vi "commander10.vi"() -> ()   [LabVIEW 2015]
uses:
  <vilib>/National Instruments/NI Dynamixel API/Dynamixel Pro Driver/Controls/Write Select Pro.ctl
  <vilib>/National Instruments/NI Dynamixel API/Dynamixel Pro Driver/Controls/Baudrate Selector.ctl
  G_LCM.vi
  G_ALL.vi
  G_SEN.vi
  <vilib>/National Instruments/NI Dynamixel API/Dynamixel Pro Driver/Write/Write Dynamixel Pro.vi
  <vilib>/National Instruments/NI Dynamixel API/Dynamixel Pro Driver/Helper VIs/Torque Disable.vi
  <vilib>/National Instruments/NI Dynamixel API/Dynamixel Pro Driver/Helper VIs/Torque Enable.vi
  <vilib>/National Instruments/NI Dynamixel API/Dynamixel Pro Driver/Dynamixel Pro Driver.lvlib
panel:
  in  "map":bool
  in  "Path Num":i32 min=0 max=4 step=1
  out "CIPV_SPEED":dbl=25.0
  out "CIPV_dist":dbl=25.0
  in  "mission":i32
  out "size(s)":i32=1381
  in  "shift torque gain":i32
  out "robotis":refnum<visa-resource-name>
  in  "y 2":dbl=1.0
  in  "y":dbl=0.5 format="%#_13g"
  in  "dist_error_gain":dbl=0.5 format="%#_13g"
  in  "Global y shift":dbl min=-5.0 max=5.0 step=0.1
  in  "d":dbl=-3.5 format="%#_13g"
  in  "car detection":bool
  in  "Velodyne":T1(ring)=enum."Velodyne 64"
  in  "reset path":bool
  in  "shifthold":dbl=0.003
  out "count":i32=100
  out "signal":picture[](array[picture])=[bytes[7530], bytes[7530], bytes[7530], bytes[7530]]
  out "sign":picture[](array[picture])=[bytes[7530], bytes[7530], bytes[7530], bytes[7530]]
  out "trafic signal ref":picture[](array[picture])=[bytes[7530], bytes[7530], bytes[7530], bytes[7530], bytes[7530], bytes[7530]]
  out "sign ref":picture[](array[picture])=[bytes[7530], bytes[7530], bytes[7530], bytes[7530], bytes[7530], bytes[7530], bytes[7530], bytes[7530], bytes[7530], bytes[7530], bytes[7530], bytes[7530], bytes[7530]]
  in  "TTL":bool=TRUE
  out "obs shift":dbl format="%.2f"
  in  "lane keep":bool
  in  "replay":bool
  in  "Global x shift":dbl min=-5.0 max=5.0 step=1.0
  out "display":u32=33
  out "control":u32=10
  in  "lane update":bool
  in  "save lcm":bool
  out "LCM Recv Data":string
  out "GPS DATA 2":T2={"type"="None", "x_lcc"=0.0, "y_lcc"=0.0, "latdev"=0.0, "londev"=0.0, "sats"=0, "gps_l1_ranges"=0, "gps_l1_mask_ranges"=0, "gps_l2_mask_ranges"=0, "Heading"=0.0, "lon"=0.0, "lat"=0.0, "time"="09:00:00.0", "hgps"=0.0, "lag"=0.0, "MAP"=""} {"lag" format="%#_5g"; "hgps" format="%#_5g"; "lat" format="%#_11g"; "lon" format="%#_11g"; "Heading" format="%#_5g"; "latdev" format="%#_4g"; "londev" format="%#_4g"}
  in  "Obs":bool
  in  "Log":bool
  out "path":u32=10
  out "sensor":u32=27 format="%02.0f"
  out "Speed limit":dbl=10.0
  out "collision":bool
  in  "Load Path":bool
  in  "Max. Vel.":dbl=10.0 min=-5.0 max=120.0 step=5.0
  out "col":i16(graph)
  out "stop":bool
  in  "Reverse":bool
  in  "STOP":bool
  out "Waveform Chart 4":cluster{"auto":i16, "run":i16}(graph)={"auto"=1, "run"=0}
  out "Waveform Chart 3":cluster{"Steer_input":dbl, dbl, "handle":dbl}(graph)={"Steer_input"=0.0, -0.0, "handle"=nan}
  out "Waveform Chart 2":T3(graph)={"VS_des"=0.0, "VS_can"=0.0, "VS_des"=10.0}
  out "Heading":cluster{"Heading":dbl, "hgps":dbl}(graph)
  out "XY Graph 2":cluster{"Y":dbl[], "Y":dbl[]}[](graph)
  out "Gauge":cluster{dbl, dbl, dbl}(knob)={0.0, 0.0, 10.0} scale=-20.0..140.0
  out "Meter":cluster{dbl, dbl, dbl}(knob)={0.0, -0.0, nan} scale=-550.0..550.0
  out "XY Graph":cluster{"Y":dbl[], "Y":dbl[]}[](graph)=[{"Y"=[], "Y"=[]}, {"Y"=[-0.0, -0.0, -0.0, -0.0, -0.0, -0.0, -0.0, -0.0, -0.0, -0.0, -0.0, -0.0, -0.0, -0.0, -0.0, -0.0, -0.0, -0.0, -0.0, -0.0, -0.0, -0.0, -0.0, -0.0, -0.0, -0.0, -0.0, -0.0, -0.0, -0.0, -0.0], "Y"=[-4.0, -3.9, -3.8, -3.7, -3.6, -3.5, -3.4, -3.3, -3.2, -3.1, -3.0, -2.9, -2.8, -2.7, -2.5999999999999996, -2.5, -2.4, -2.3, -2.2, -2.0999999999999996, -2.0, -1.9, -1.7999999999999998, -1.6999999999999997, -1.5999999999999996, -1.5, -1.4, -1.2999999999999998, -1.1999999999999997, -1.0999999999999996, -1.0]}, {"Y"=[0.0], "Y"=[0.0]}, {"Y"=[], "Y"=[]}, {"Y"=[-0.925, -0.925, -0.925, -0.6775, -0.6775, -0.925, -0.925, -0.925, -0.925, -0.6775, -0.6775, -0.925, -0.925, -0.925, 0.9025, 0.9025, 0.9025, 0.6775, 0.6775, 0.9025, 0.9025, 0.9025, 0.9025, 0.6775, 0.6775, 0.9025, 0.9025, 0.9025, -0.925], "Y"=[-0.75, -0.224, 0.224, 0.224, -0.224, -0.224, 0.224, 2.415, 2.885, 2.885, 2.415, 2.415, 2.885, 3.5, 3.5, 2.885, 2.415, 2.415, 2.885, 2.885, 2.415, 0.224, -0.224, -0.224, 0.224, 0.224, -0.224, -0.75, -0.75]}, {"Y"=[-0.11693930899008871, -0.11530935243371389, -0.11366872898963808, -0.11201743865786128, -0.11035548143838347, -0.10868285733120467, -0.10699956633632488, -0.10530560845374409, -0.1036009836834623, -0.10188569202547951, -0.10015973347979573, -0.09842310804641094, -0.09667581572532517, -0.09491785651653842, -0.09314923042005063, -0.09136993743586189, -0.08957997756397212, -0.08777935080438137, -0.08596805715708963, -0.08414609662209688, -0.08231346919940313, -0.0804701748890084, -0.07861621369091265, -0.07675158560511593, -0.07487629063161819, -0.07299032877041947, -0.07109370002151975, -0.06918640438491905, -0.06726844186061733, -0.06533981244861461, -0.06340051614891093, -0.061450552961506213, -0.05948992288640052, -0.05751862592359382, -0.055536662073086135, -0.05354403133487746, -0.05154073370896778, -0.0495267691953571, -0.04750213779404542, -0.045466839505032754, -0.04342087432831909, -0.04136424226390442, -0.03929694331178877, -0.03721897747197212, -0.035130344744454464, -0.033031045129235825, -0.03092107862631617, -0.028800445235695537, -0.02666914495737389, -0.024527177791351266, -0.02237454373762765, -0.02021124279620301, -0.018037274967077403, -0.015852640250250776, -0.013657338645723171, -0.011451370153494574, -0.009234734773564957, -0.007007432505934365, -0.004769463350602757, -0.002520827307570167, -0.0002615243768365888, 0.0020084454415980058, 0.004289082147733582, 0.0065803857415701675, 0.008882356223107735, 0.011194993592346297, 0.013518297849285876, 0.01585226899392643, 0.018196907026268, 0.020552211946310545, 0.02291818375405409, 0.025294822449498655, 0.02768212803264418, 0.03008010050349072, 0.03248873986203825, 0.03490804610828678, 0.037338019242236314, 0.03977865926388684, 0.04222996617323836, 0.044691939970290875, 0.04716458065504438, 0.04964788822749888, 0.05214186268765442, 0.05464650403551091, 0.057161812271068396, 0.05968778739432688, 0.06222442940528636, 0.06477173830394688, 0.06732971409030836, 0.06989835676437083, 0.07247766632613428, 0.07506764277559874, 0.07766828611276426, 0.08027959633763071, 0.08290157345019813, 0.08553421745046658, 0.08817752833843606, 0.09083150611410651, 0.09349615077747794, 0.09617146232855037, 0.0988574407673238], "Y"=[-4.0, -3.9, -3.8, -3.7, -3.6, -3.5, -3.4, -3.3, -3.2, -3.1, -3.0, -2.9, -2.8, -2.7, -2.5999999999999996, -2.5, -2.4, -2.3, -2.2, -2.0999999999999996, -2.0, -1.9, -1.7999999999999998, -1.6999999999999997, -1.5999999999999996, -1.5, -1.4, -1.2999999999999998, -1.1999999999999997, -1.0999999999999996, -1.0, -0.8999999999999999, -0.7999999999999998, -0.6999999999999997, -0.5999999999999996, -0.5, -0.3999999999999999, -0.2999999999999998, -0.19999999999999973, -0.09999999999999964, 0.0, 0.10000000000000053, 0.20000000000000018, 0.2999999999999998, 0.40000000000000036, 0.5, 0.6000000000000005, 0.7000000000000002, 0.8000000000000007, 0.9000000000000004, 1.0, 1.1000000000000005, 1.2000000000000002, 1.3000000000000007, 1.4000000000000004, 1.5, 1.6000000000000005, 1.7000000000000002, 1.8000000000000007, 1.9000000000000004, 2.0, 2.1000000000000005, 2.2, 2.3000000000000007, 2.4000000000000004, 2.5, 2.6000000000000005, 2.7, 2.8000000000000007, 2.9000000000000004, 3.0, 3.1000000000000005, 3.2, 3.3000000000000007, 3.4000000000000004, 3.5, 3.6000000000000005, 3.7, 3.8000000000000007, 3.9000000000000004, 4.0, 4.1, 4.200000000000001, 4.300000000000001, 4.4, 4.5, 4.6, 4.700000000000001, 4.800000000000001, 4.9, 5.0, 5.1, 5.200000000000001, 5.300000000000001, 5.4, 5.5, 5.600000000000001, 5.700000000000001, 5.800000000000001, 5.9, 6.0]}, {"Y"=[0.8254985256386238, 0.8528194590155173, 0.8796538166129886, 0.9060015984310377, 0.9318628044696647, 0.9572374347288698, 0.9821254892086528, 1.0065269679090136, 1.0304418708299523, 1.0538701979714689, 1.0768119493335635, 1.099267124916236, 1.1212357247194864, 1.1427177487433147, 1.163713196987721, 1.184222069452705, 1.204244366138267, 1.2237800870444069, 1.2428292321711245, 1.2613918015184205, 1.279467795086294, 1.2970572128747455, 1.314160054883775, 1.3307763211133825, 1.3469060115635676, 1.3625491262343308, 1.3777056651256718, 1.392375628237591, 1.4065590155700878, 1.4202558271231627, 1.4334660628968152, 1.4461897228910459, 1.4584268071058544, 1.4701773155412408, 1.4814412481972052, 1.4922186050737474, 1.5025093861708676, 1.5123135914885657, 1.5216312210268417, 1.5304622747856955, 1.5388067527651272, 1.546664654965137, 1.5540359813857245, 1.56092073202689, 1.5673189068886335, 1.5732305059709548, 1.578655529273854, 1.583593976797331, 1.5880458485413862, 1.592011144506019, 1.5954898646912299, 1.5984820090970187, 1.6009875777233853, 1.60300657057033, 1.6045389876378524, 1.605584828925953, 1.606144094434631, 1.6062167841638872, 1.6058028981137213, 1.6049024362841335, 1.6035153986751234, 1.601641785286691, 1.599281596118837, 1.5964348311715606, 1.5931014904448622, 1.5892815739387416, 1.584975081653199, 1.5801820135882343, 1.5749023697438473, 1.5691361501200385, 1.5628833547168075, 1.5561439835341544, 1.5489180365720792, 1.541205513830582, 1.5330064153096625, 1.5243207410093211, 1.5151484909295576, 1.505489665070372, 1.4953442634317642, 1.4847122860137343, 1.4735937328162825, 1.4619886038394085, 1.4498968990831123, 1.437318618547394, 1.4242537622322538, 1.4107023301376915, 1.396664322263707, 1.3821397386103003, 1.3671285791774717, 1.351630843965221, 1.335646532973548, 1.3191756462024533, 1.302218183651936, 1.284774145321997, 1.2668435312126356, 1.2484263413238526, 1.229522575655647, 1.2101322342080194, 1.19025531698097, 1.1698918239744982, 1.1490417551886045], "Y"=[-4.0, -3.9, -3.8, -3.7, -3.6, -3.5, -3.4, -3.3, -3.2, -3.1, -3.0, -2.9, -2.8, -2.7, -2.5999999999999996, -2.5, -2.4, -2.3, -2.2, -2.0999999999999996, -2.0, -1.9, -1.7999999999999998, -1.6999999999999997, -1.5999999999999996, -1.5, -1.4, -1.2999999999999998, -1.1999999999999997, -1.0999999999999996, -1.0, -0.8999999999999999, -0.7999999999999998, -0.6999999999999997, -0.5999999999999996, -0.5, -0.3999999999999999, -0.2999999999999998, -0.19999999999999973, -0.09999999999999964, 0.0, 0.10000000000000053, 0.20000000000000018, 0.2999999999999998, 0.40000000000000036, 0.5, 0.6000000000000005, 0.7000000000000002, 0.8000000000000007, 0.9000000000000004, 1.0, 1.1000000000000005, 1.2000000000000002, 1.3000000000000007, 1.4000000000000004, 1.5, 1.6000000000000005, 1.7000000000000002, 1.8000000000000007, 1.9000000000000004, 2.0, 2.1000000000000005, 2.2, 2.3000000000000007, 2.4000000000000004, 2.5, 2.6000000000000005, 2.7, 2.8000000000000007, 2.9000000000000004, 3.0, 3.1000000000000005, 3.2, 3.3000000000000007, 3.4000000000000004, 3.5, 3.6000000000000005, 3.7, 3.8000000000000007, 3.9000000000000004, 4.0, 4.1, 4.200000000000001, 4.300000000000001, 4.4, 4.5, 4.6, 4.700000000000001, 4.800000000000001, 4.9, 5.0, 5.1, 5.200000000000001, 5.300000000000001, 5.4, 5.5, 5.600000000000001, 5.700000000000001, 5.800000000000001, 5.9, 6.0]}, {"Y"=[-1.0593771436188013, -1.0834381638829451, -1.1069912745922648, -1.1300364757467602, -1.1525737673464316, -1.1746031493912792, -1.1961246218813026, -1.2171381848165017, -1.2376438381968768, -1.257641582022428, -1.277131416293155, -1.296113341009058, -1.314587356170137, -1.3325534617763914, -1.3500116578278223, -1.3669619443244287, -1.3834043212662113, -1.3993387886531696, -1.4147653464853038, -1.4296839947626143, -1.4440947334851004, -1.4579975626527624, -1.4713924822656004, -1.4842794923236142, -1.4966585928268041, -1.5085297837751699, -1.5198930651687115, -1.530748437007429, -1.5410958992913224, -1.5509354520203917, -1.5602670951946371, -1.5690908288140584, -1.5774066528786554, -1.5852145673884286, -1.5925145723433776, -1.5993066677435024, -1.605590853588803, -1.6113671298792798, -1.6166354966149326, -1.621395953795761, -1.6256485014217654, -1.6293931394929457, -1.632629868009302, -1.6353586869708343, -1.6375795963775424, -1.6392925962294265, -1.6404976865264864, -1.6411948672687222, -1.6413841384561338, -1.6410655000887215, -1.6402389521664853, -1.6389044946894247, -1.6370621276575401, -1.6347118510708316, -1.6318536649292987, -1.628487569232942, -1.624613563981761, -1.620231649175756, -1.615341824814927, -1.6099440908992737, -1.6040384474287965, -1.5976248944034952, -1.5907034318233697, -1.5832740596884203, -1.5753367779986467, -1.566891586754049, -1.5579384859546273, -1.5484774756003814, -1.5385085556913114, -1.5280317262274175, -1.5170469872086993, -1.505554338635157, -1.4935537805067909, -1.4810453128236005, -1.4680289355855862, -1.4545046487927475, -1.440472452445085, -1.4259323465425984, -1.4108843310852874, -1.3953284060731526, -1.3792645715061937, -1.3626928273844108, -1.3456131737078034, -1.3280256104763721, -1.309930137690117, -1.2913267553490377, -1.2722154634531344, -1.2525962620024065, -1.232469150996855, -1.2118341304364795, -1.1906912003212795, -1.1690403606512558, -1.1468816114264073, -1.1242149526467355, -1.1010403843122396, -1.077357906422919, -1.0531675189787748, -1.0284692219798064, -1.0032630154260138, -0.9775488993173974, -0.9513268736539569], "Y"=[-4.0, -3.9, -3.8, -3.7, -3.6, -3.5, -3.4, -3.3, -3.2, -3.1, -3.0, -2.9, -2.8, -2.7, -2.5999999999999996, -2.5, -2.4, -2.3, -2.2, -2.0999999999999996, -2.0, -1.9, -1.7999999999999998, -1.6999999999999997, -1.5999999999999996, -1.5, -1.4, -1.2999999999999998, -1.1999999999999997, -1.0999999999999996, -1.0, -0.8999999999999999, -0.7999999999999998, -0.6999999999999997, -0.5999999999999996, -0.5, -0.3999999999999999, -0.2999999999999998, -0.19999999999999973, -0.09999999999999964, 0.0, 0.10000000000000053, 0.20000000000000018, 0.2999999999999998, 0.40000000000000036, 0.5, 0.6000000000000005, 0.7000000000000002, 0.8000000000000007, 0.9000000000000004, 1.0, 1.1000000000000005, 1.2000000000000002, 1.3000000000000007, 1.4000000000000004, 1.5, 1.6000000000000005, 1.7000000000000002, 1.8000000000000007, 1.9000000000000004, 2.0, 2.1000000000000005, 2.2, 2.3000000000000007, 2.4000000000000004, 2.5, 2.6000000000000005, 2.7, 2.8000000000000007, 2.9000000000000004, 3.0, 3.1000000000000005, 3.2, 3.3000000000000007, 3.4000000000000004, 3.5, 3.6000000000000005, 3.7, 3.8000000000000007, 3.9000000000000004, 4.0, 4.1, 4.200000000000001, 4.300000000000001, 4.4, 4.5, 4.6, 4.700000000000001, 4.800000000000001, 4.9, 5.0, 5.1, 5.200000000000001, 5.300000000000001, 5.4, 5.5, 5.600000000000001, 5.700000000000001, 5.800000000000001, 5.9, 6.0]}, {"Y"=[], "Y"=[]}, {"Y"=[0.0], "Y"=[0.0]}, {"Y"=[], "Y"=[]}, {"Y"=[], "Y"=[]}, {"Y"=[0.0], "Y"=[0.0]}, {"Y"=[-2.34, -2.34, -2.34, -2.34, -2.2800000000000002, -2.2800000000000002, -2.2800000000000002, -2.2800000000000002, -2.22, -2.22, -2.22, -2.16, -2.16, -2.16, -2.1, -2.1, -2.1, -2.04, -2.04, -2.04, -2.04, -1.98, -1.98, -1.98, -1.98, -1.68, -1.68, -1.68, -1.68, -1.68, -1.68, -1.68, -1.68, -1.68, -1.68, -1.68, -1.68, -1.68, -1.68, -1.68, -1.68, -1.68, -1.68, -1.68, -1.68, -1.68, -1.68, -1.68, -1.68, -1.68, -1.68, -1.68, -1.68, -1.68, -1.68, -1.68, -1.68, -1.68, -1.68, -1.68, -1.68, -1.68, -1.68, -1.68, -1.68, -1.68, -1.68, -1.62, -1.62, -1.62, -1.62, -1.62, -1.62, -1.62, -1.62, -1.62, -1.62, -1.62, -1.62, -1.62, -1.62, -1.62, -1.62, -1.62, -1.62, -1.62, -1.62, -1.62, -1.62, -1.62, -1.62, -1.62, -1.62, -1.62, -1.62, -1.62, -1.62, -1.62, -1.62, -1.62, -1.62, -1.62, -1.62, -1.62, -1.62, -1.62, -1.62, -1.62, -1.62, -1.62, -1.62, -1.62, -1.62, -1.62, -1.62, -1.62, -1.62, -1.62, -1.62, -1.62, -1.62, -1.62, -1.62, -1.62, -1.62, -1.62, -1.62, -1.62, -1.62, -1.62, -1.62, -1.62, -1.62, -1.62, -1.62, -1.62, -1.62, -1.62, -1.62, -1.62, -1.62, -1.62, -1.62, -1.62, -1.62, -1.62, -1.62, -1.56, -1.56, -1.56, -1.56, -1.56, -1.56, -1.56, -1.56, -1.56, -1.56, -1.56, -1.56, -1.56, -1.56, -1.56, -1.56, -1.56, -1.56, -1.56, -1.56, -1.56, -1.56, -1.56, -1.56, -1.56, -1.56, -1.56, -1.56, -1.56, -1.56, -1.56, -1.56, -1.56, -1.56, -1.56, -1.56, -1.56, -1.56, -1.56, -1.56, -1.56, -1.56, -1.56, -1.56, -1.56, -1.56, -1.56, -1.56, -1.56, -1.56, -1.56, -1.56, -1.56, -1.56, -1.56, -1.56, -1.56, -1.56, -1.56, -1.56, -1.56, -1.56, -1.56, -1.56, -1.56, -1.56, -1.56, -1.56, -1.56, -1.56, -1.56, -1.56, -1.56, -1.56, -1.56, -1.56, -1.56, -1.56, -1.56, -1.56, -1.56, -1.56, -1.56, -1.56, -1.56, -1.56, -1.56, -1.56, -1.56, -1.56, -1.56, -1.56, -1.56, -1.56, -1.5, -1.5, -1.5, -1.5, -1.5, -1.5, -1.5, -1.5, -1.5, -1.5, -1.5, -1.5, -1.5, -1.5, -1.5, -1.5, -1.5, -1.5, -1.5, -1.5, -1.5, -1.5, -1.5, -1.5, -1.5, -1.5, -1.5, -1.5, -1.5, -1.5, -1.5, -1.5, -1.5, -1.5, -1.5, -1.5, -1.5, -1.5, -1.5, -1.5, -1.5, -1.5, -1.5, -1.5, -1.5, -1.5, -1.5, -1.5, -1.5, -1.5, -1.44, -1.44, -1.44, -1.44, -1.44, -1.44, -1.44, -1.44, -1.44, -1.44, -1.44, -1.44, -1.44, -1.44, -1.44, -1.44, -1.44, -1.44, -1.44, -1.44, -1.44, -1.44, -1.44, -1.44, -1.44, -1.44, -1.44, -1.44, -1.44, -1.44, -1.44, -1.44, -1.44, -1.44, -1.3800000000000001, -1.3800000000000001, -1.3800000000000001, -1.3800000000000001, -1.3800000000000001, -1.3800000000000001, -1.3800000000000001, -1.3800000000000001, -1.3800000000000001, -1.3800000000000001, -1.3800000000000001, -1.3800000000000001, -1.3800000000000001, -1.3800000000000001, -1.3800000000000001, -1.3800000000000001, -1.3800000000000001, -1.3800000000000001, -1.3800000000000001, -1.3800000000000001, -1.3800000000000001, -1.32, -1.32, -1.32, -1.32, -1.32, -1.32, -1.32, -1.32, -1.32, -1.32, -1.32, -1.32, -1.32, -1.32, -1.32, -1.32, -1.32, -1.32, -1.32, -1.32, -1.32, -1.26, -1.26, -1.26, -1.26, -1.26, -1.26, -1.26, -1.26, -1.26, -1.26, -1.26, -1.26, -1.26, -1.26, -1.26, -1.26, -1.26, -1.26, -1.26, -1.26, -1.26, -1.26, -1.26, -1.26, -1.26, -1.26, -1.26, -1.26, -1.2, -1.2, -1.2, -1.2, -1.2, -1.2, -1.2, -1.2, -1.2, -1.2, -1.2, -1.2, -1.2, -1.2, -1.2, -1.2, -1.2, -1.2, -1.2, -1.2, -1.2, -1.2, -1.2, -1.2, -1.2, -1.2, -1.2, -1.2, -1.2, -1.1400000000000001, -1.1400000000000001, -1.1400000000000001, -1.1400000000000001, -1.1400000000000001, -1.1400000000000001, -1.1400000000000001, -1.1400000000000001, -1.1400000000000001, -1.1400000000000001, -1.1400000000000001, -1.1400000000000001, -1.1400000000000001, -1.1400000000000001, -1.1400000000000001, -1.1400000000000001, -1.1400000000000001, -1.1400000000000001, -1.1400000000000001, -1.1400000000000001, -1.1400000000000001, -1.1400000000000001, -1.1400000000000001, -1.1400000000000001, -1.1400000000000001, -1.1400000000000001, -1.1400000000000001, -1.08, -1.08, -1.08, -1.08, -1.08, -1.08, -1.08, -1.08, -1.08, -1.08, -1.08, -1.08, -1.08, -1.08, -1.08, -1.08, -1.08, -1.08, -1.08, -1.08, -1.08, -1.02, -1.02, -1.02, -1.02, -1.02, -1.02, -1.02, -1.02, -1.02, -1.02, -1.02, -1.02, -1.02, -1.02, -1.02, -1.02, -1.02, -1.02, -1.02, -1.02, -0.96, -0.96, -0.96, -0.96, -0.96, -0.96, -0.96, -0.96, -0.96, -0.96, -0.96, -0.96, -0.96, -0.96, -0.96, -0.96, -0.96, -0.96, -0.96, -0.96, -0.96, -0.96, -0.96, -0.96, -0.96, -0.96, -0.9, -0.9, -0.9, -0.9, -0.9, -0.9, -0.9, -0.9, -0.9, -0.9, -0.9, -0.9, -0.9, -0.9, -0.9, -0.9, -0.9, -0.9, -0.9, -0.9, -0.9, -0.9, -0.9, -0.9, -0.9, -0.9, -0.9, -0.84, -0.84, -0.84, -0.84, -0.84, -0.84, -0.84, -0.84, -0.84, -0.84, -0.84, -0.84, -0.84, -0.84, -0.84, -0.84, -0.84, -0.84, -0.84, -0.84, -0.84, -0.84, -0.84, -0.84, -0.84, -0.84, -0.84, -0.78, -0.78, -0.78, -0.78, -0.78, -0.78, -0.78, -0.78, -0.78, -0.78, -0.78, -0.78, -0.78, -0.78, -0.78, -0.78, -0.78, -0.78, -0.78, -0.78, -0.78, -0.78, -0.78, -0.78, -0.72, -0.72, -0.72, -0.72, -0.72, -0.72, -0.72, -0.72, -0.72, -0.72, -0.72, -0.72, -0.72, -0.72, -0.72, -0.72, -0.72, -0.72, -0.72, -0.72, -0.72, -0.72, -0.66, -0.66, -0.66, -0.66, -0.66, -0.66, -0.66, -0.66, -0.66, -0.66, -0.66, -0.66, -0.66, -0.66, -0.66, -0.66, -0.66, -0.66, -0.66, -0.66, -0.66, -0.66, -0.66, -0.66, -0.66, -0.66, -0.66, -0.66, -0.66, -0.66, -0.66, -0.66, -0.66, -0.66, -0.6, -0.6, -0.6, -0.6, -0.6, -0.6, -0.6, -0.6, -0.6, -0.6, -0.6, -0.6, -0.6, -0.6, -0.6, -0.6, -0.6, -0.6, -0.6, -0.6, -0.6, -0.6, -0.6, -0.6, -0.6, -0.6, -0.6, -0.54, -0.54, -0.54, -0.54, -0.54, -0.54, -0.54, -0.54, -0.54, -0.54, -0.54, -0.54, 0.54, 0.54, 0.54, 0.54, 0.54, 0.54, 0.54, 0.54, 0.54, 0.6, 0.6, 0.6, 0.6, 0.6, 0.6, 0.6, 0.6, 0.6, 0.6, 0.6, 0.6, 0.6, 0.66, 0.66, 0.66, 0.66, 0.66, 0.66, 0.66, 0.66, 0.66, 0.66, 0.66, 0.66, 0.66, 0.66, 0.72, 0.72, 0.72, 0.72, 0.72, 0.72, 0.72, 0.72, 0.72, 0.78, 0.78, 0.78, 0.78, 0.78, 0.78, 0.78, 0.78, 0.78, 0.78, 0.78, 0.78, 0.84, 0.84, 0.84, 0.84, 0.84, 0.84, 0.84, 0.84, 0.84, 0.84, 0.84, 0.84, 0.9, 0.9, 0.9, 0.9, 0.9, 0.9, 0.9, 0.9, 0.9, 0.9, 0.9, 0.9, 0.9, 0.9, 0.9, 0.9, 0.9, 0.9, 0.9, 0.9, 0.96, 0.96, 0.96, 0.96, 0.96, 0.96, 0.96, 0.96, 0.96, 0.96, 0.96, 0.96, 0.96, 0.96, 0.96, 0.96, 0.96, 0.96, 0.96, 0.96, 0.96, 0.96, 0.96, 0.96, 0.96, 0.96, 0.96, 0.96, 1.02, 1.02, 1.02, 1.02, 1.02, 1.02, 1.02, 1.02, 1.02, 1.02, 1.02, 1.02, 1.02, 1.02, 1.02, 1.02, 1.02, 1.02, 1.02, 1.02, 1.02, 1.02, 1.02, 1.02, 1.02, 1.02, 1.02, 1.02, 1.02, 1.02, 1.02, 1.02, 1.08, 1.08, 1.08, 1.08, 1.08, 1.08, 1.08, 1.08, 1.08, 1.08, 1.08, 1.08, 1.08, 1.08, 1.08, 1.08, 1.08, 1.08, 1.08, 1.08, 1.08, 1.08, 1.08, 1.08, 1.08, 1.08, 1.08, 1.08, 1.08, 1.08, 1.08, 1.08, 1.08, 1.08, 1.08, 1.08, 1.1400000000000001, 1.1400000000000001, 1.1400000000000001, 1.1400000000000001, 1.1400000000000001, 1.1400000000000001, 1.1400000000000001, 1.1400000000000001, 1.1400000000000001, 1.1400000000000001, 1.1400000000000001, 1.1400000000000001, 1.1400000000000001, 1.1400000000000001, 1.1400000000000001, 1.1400000000000001, 1.1400000000000001, 1.1400000000000001, 1.1400000000000001, 1.1400000000000001, 1.1400000000000001, 1.1400000000000001, 1.1400000000000001, 1.1400000000000001, 1.1400000000000001, 1.1400000000000001, 1.1400000000000001, 1.1400000000000001, 1.1400000000000001, 1.1400000000000001, 1.1400000000000001, 1.1400000000000001, 1.1400000000000001, 1.1400000000000001, 1.1400000000000001, 1.1400000000000001, 1.1400000000000001, 1.2, 1.2, 1.2, 1.2, 1.2, 1.2, 1.2, 1.2, 1.2, 1.2, 1.2, 1.2, 1.2, 1.2, 1.2, 1.2, 1.2, 1.2, 1.2, 1.2, 1.2, 1.2, 1.2, 1.2, 1.2, 1.2, 1.2, 1.2, 1.2, 1.26, 1.26, 1.26, 1.26, 1.26, 1.26, 1.26, 1.26, 1.26, 1.26, 1.26, 1.26, 1.26, 1.26, 1.26, 1.26, 1.26, 1.26, 1.26, 1.26, 1.26, 1.26, 1.26, 1.26, 1.26, 1.26, 1.26, 1.26, 1.26, 1.26, 1.26, 1.26, 1.26, 1.26, 1.32, 1.32, 1.32, 1.32, 1.32, 1.32, 1.32, 1.32, 1.32, 1.32, 1.32, 1.32, 1.32, 1.32, 1.32, 1.32, 1.32, 1.32, 1.32, 1.32, 1.32, 1.32, 1.32, 1.32, 1.32, 1.32, 1.32, 1.32, 1.32, 1.32, 1.32, 1.32, 1.32, 1.32, 1.32, 1.3800000000000001, 1.3800000000000001, 1.3800000000000001, 1.3800000000000001, 1.3800000000000001, 1.3800000000000001, 1.3800000000000001, 1.3800000000000001, 1.3800000000000001, 1.3800000000000001, 1.3800000000000001, 1.3800000000000001, 1.3800000000000001, 1.3800000000000001, 1.3800000000000001, 1.3800000000000001, 1.3800000000000001, 1.3800000000000001, 1.3800000000000001, 1.3800000000000001, 1.3800000000000001, 1.3800000000000001, 1.3800000000000001, 1.3800000000000001, 1.3800000000000001, 1.3800000000000001, 1.3800000000000001, 1.3800000000000001, 1.3800000000000001, 1.3800000000000001, 1.3800000000000001, 1.3800000000000001, 1.3800000000000001, 1.3800000000000001, 1.3800000000000001, 1.44, 1.44, 1.44, 1.44, 1.44, 1.44, 1.44, 1.44, 1.44, 1.44, 1.44, 1.44, 1.44, 1.44, 1.44, 1.44, 1.44, 1.44, 1.44, 1.44, 1.44, 1.44, 1.44, 1.44, 1.44, 1.44, 1.44, 1.44, 1.44, 1.44, 1.44, 1.44, 1.44, 1.44, 1.44, 1.44, 1.44, 1.44, 1.44, 1.44, 1.5, 1.5, 1.5, 1.5, 1.5, 1.5, 1.5, 1.5, 1.5, 1.5, 1.5, 1.5, 1.5, 1.5, 1.5, 1.5, 1.5, 1.5, 1.5, 1.5, 1.5, 1.5, 1.5, 1.5, 1.5, 1.5, 1.5, 1.5, 1.5, 1.5, 1.5, 1.5, 1.5, 1.5, 1.5, 1.5, 1.5, 1.5, 1.5, 1.5, 1.5, 1.5, 1.5, 1.5, 1.5, 1.5, 1.5, 1.5, 1.5, 1.5, 1.5, 1.5, 1.5, 1.5, 1.5, 1.5, 1.5, 1.5, 1.5, 1.5, 1.5, 1.5, 1.5, 1.56, 1.56, 1.56, 1.56, 1.56, 1.56, 1.56, 1.56, 1.56, 1.56, 1.56, 1.56, 1.56, 1.56, 1.56, 1.56, 1.56, 1.56, 1.56, 1.56, 1.56, 1.56, 1.56, 1.56, 1.56, 1.56, 1.56, 1.56, 1.56, 1.56, 1.56, 1.56, 1.56, 1.56, 1.56, 1.56, 1.56, 1.56, 1.56, 1.56, 1.56, 1.56, 1.56, 1.56, 1.56, 1.56, 1.56, 1.56, 1.56, 1.56, 1.56, 1.56, 1.56, 1.56, 1.56, 1.56, 1.56, 1.56, 1.56, 1.56, 1.56, 1.56, 1.56, 1.56, 1.56, 1.56, 1.56, 1.56, 1.56, 1.56, 1.56, 1.56, 1.56, 1.56, 1.56, 1.56, 1.56, 1.56, 1.56, 1.56, 1.56, 1.56, 1.56, 1.56, 1.56, 1.62, 1.62, 1.62, 1.62, 1.62, 1.62, 1.62, 1.62, 1.62, 1.62, 1.62, 1.62, 1.62, 1.62, 1.62, 1.62, 1.62, 1.62, 1.62, 1.62, 1.62, 1.62, 1.62, 1.62, 1.62, 1.62, 1.62, 1.62, 1.62, 1.62, 1.62, 1.62, 1.62, 1.62, 1.62, 1.62, 1.62, 1.62, 1.62, 1.62, 1.62, 1.62, 1.62, 1.62, 1.62, 1.62, 1.62, 1.62, 1.62, 1.62, 1.62, 1.62, 1.62, 1.62, 1.62, 1.62, 1.62, 1.62, 1.62, 1.62, 1.62, 1.62, 1.62, 1.62, 1.62, 1.62, 1.62, 1.62, 1.62, 1.62, 1.62, 1.62, 1.68, 1.68, 1.68, 1.68, 1.68, 1.68, 1.68, 1.68, 1.68, 1.68, 1.68, 1.68, 1.68, 1.68, 1.74, 1.74, 1.74, 1.74, 1.74, 1.8, 1.8, 1.8, 1.8, 1.8, 1.8, 1.86, 1.86, 1.86, 1.86, 1.92, 1.92, 1.92, 1.92, 1.92, 1.98, 1.98, 1.98, 1.98, 1.98, 1.98, 2.04, 2.04, 2.04, 2.04, 2.04, 2.1, 2.1, 2.1, 2.1, 2.1, 2.16, 2.16, 2.16, 2.16, 2.22, 2.22, 2.22, 2.22, 2.2800000000000002, 2.2800000000000002, 2.2800000000000002, 2.2800000000000002, 2.2800000000000002, 2.2800000000000002, 2.2800000000000002, 2.34, 2.34, 2.34, 2.34, 2.34, 2.34, 2.34, 2.34, 2.34, 2.34], "Y"=[-5.88, -5.94, -6.0, -6.0600000000000005, -5.88, -5.94, -6.0, -6.0600000000000005, -5.88, -5.94, -6.0, -6.3, -6.36, -6.42, -6.3, -6.36, -6.42, -6.24, -6.3, -6.36, -6.42, -6.24, -6.3, -6.36, -6.42, 2.04, 1.98, 1.92, 1.86, 1.8, 1.74, 1.68, 1.62, 1.56, 1.5, 1.3800000000000001, 1.32, 1.26, 1.2, 1.1400000000000001, 1.08, 1.02, 0.96, 0.9, 0.84, 0.78, 0.72, 0.66, 0.6, 0.54, 0.48, 0.42, 0.36, 0.3, 0.24, 0.18, 0.12, 0.06, -0.0, -0.06, -0.12, -0.18, -0.24, -0.3, -0.36, -0.42, -0.48, 3.24, 3.18, 3.12, 3.06, 3.0, 2.94, 2.88, 2.82, 2.7600000000000002, 2.7, 2.64, 2.58, 2.52, 2.46, 2.4, 2.34, 2.2800000000000002, 2.22, 2.16, 2.1, 2.04, 1.98, 1.92, 1.86, 1.8, 1.74, 1.68, 1.62, 1.56, 1.5, 1.44, 1.3800000000000001, 1.32, 1.26, 1.2, 1.1400000000000001, 1.08, 1.02, 0.96, 0.9, 0.84, 0.78, 0.72, 0.66, 0.6, 0.54, 0.48, 0.42, 0.36, 0.3, 0.24, 0.18, 0.12, 0.06, -0.0, -0.06, -0.12, -0.18, -0.24, -0.3, -0.36, -0.42, -0.48, -0.54, -0.6, -0.66, -0.72, -0.78, -0.84, -0.9, -0.96, -1.02, -1.08, -1.1400000000000001, -1.2, -1.26, -1.32, -1.3800000000000001, -1.44, -1.5, 3.72, 3.66, 3.6, 3.54, 3.48, 3.42, 3.36, 3.3000000000000003, 3.24, 3.18, 3.12, 3.06, 3.0, 2.94, 2.88, 2.82, 2.7600000000000002, 2.7, 2.64, 2.58, 2.52, 2.46, 2.4, 2.34, 2.2800000000000002, 2.22, 2.16, 2.1, 2.04, 1.98, 1.92, 1.86, 1.8, 1.74, 1.68, 1.62, 1.56, 1.5, 1.44, 1.3800000000000001, 1.32, 1.26, 1.2, 1.1400000000000001, 1.08, 1.02, 0.96, 0.9, 0.84, 0.78, 0.72, 0.66, 0.6, 0.54, 0.48, 0.42, 0.36, 0.3, 0.24, 0.18, 0.12, 0.06, -0.0, -0.06, -0.12, -0.18, -0.24, -0.3, -0.36, -0.42, -0.48, -0.54, -0.6, -0.66, -0.72, -0.78, -0.84, -0.9, -0.96, -1.02, -1.08, -1.1400000000000001, -1.2, -1.26, -1.32, -1.3800000000000001, -1.44, -1.5, -1.56, -1.62, -1.68, -1.74, -1.8, -1.86, 3.72, 3.66, 3.6, 3.54, 3.48, 3.42, 3.36, 3.3000000000000003, 3.24, 3.18, 3.12, 3.06, 3.0, 2.94, 2.88, 2.82, 2.7600000000000002, 2.7, 2.64, 2.58, 2.52, 2.46, 2.4, 2.34, -0.54, -0.6, -0.66, -0.84, -0.9, -0.96, -1.02, -1.08, -1.1400000000000001, -1.2, -1.26, -1.32, -1.3800000000000001, -1.44, -1.5, -1.56, -1.62, -1.68, -1.74, -1.8, -1.86, -1.92, -1.98, -2.04, -2.1, -2.16, 3.96, 3.9, 3.84, 3.7800000000000002, 3.72, 3.66, 3.6, 3.54, 3.48, 3.42, 3.36, 3.3000000000000003, 3.24, 3.18, 3.12, -1.44, -1.5, -1.56, -1.62, -1.68, -1.74, -1.8, -1.86, -1.92, -1.98, -2.04, -2.1, -2.16, -2.22, -2.2800000000000002, -2.34, -2.4, -2.46, -2.52, 4.2, 4.14, 4.08, 4.0200000000000005, 3.96, 3.9, 3.84, 3.7800000000000002, 3.72, 3.66, -1.98, -2.04, -2.1, -2.16, -2.22, -2.2800000000000002, -2.34, -2.4, -2.46, -2.52, -2.58, 4.5600000000000005, 4.5, 4.44, 4.38, 4.32, 4.26, 4.2, 4.14, 4.08, 4.0200000000000005, 3.96, -2.34, -2.4, -2.46, -2.52, -2.58, -2.64, -2.7, -2.7600000000000002, -2.82, -2.88, 4.92, 4.86, 4.8, 4.74, 4.68, 4.62, 4.5600000000000005, 4.5, 4.44, 4.38, 4.32, 4.26, 4.2, -2.52, -2.58, -2.64, -2.7, -2.7600000000000002, -2.82, -2.88, -2.94, -3.0, -3.06, -3.12, -3.18, -3.24, -3.3000000000000003, -3.36, 5.16, 5.1000000000000005, 5.04, 4.98, 4.92, 4.86, 4.8, 4.74, 4.68, 4.62, 4.5600000000000005, 4.5, 4.44, 4.38, -2.94, -3.0, -3.06, -3.12, -3.18, -3.24, -3.3000000000000003, -3.36, -3.42, -3.48, -3.54, -3.6, -3.66, -3.72, -3.7800000000000002, 5.64, 5.58, 5.5200000000000005, 5.46, 5.4, 5.34, 5.28, 5.22, 5.16, 5.1000000000000005, 5.04, 4.98, 4.92, 4.86, 4.8, -3.36, -3.42, -3.48, -3.54, -3.6, -3.66, -3.72, -3.7800000000000002, -3.84, -3.9, -3.96, -4.0200000000000005, 6.0, 5.94, 5.88, 5.82, 5.76, 5.7, 5.64, 5.58, 5.5200000000000005, 5.46, 5.4, 5.34, 5.28, 5.22, -3.84, -3.9, -3.96, -4.0200000000000005, -4.08, -4.14, -4.2, 6.24, 6.18, 6.12, 6.0600000000000005, 6.0, 5.94, 5.88, 5.82, 5.76, 5.7, 5.64, 5.58, 5.5200000000000005, -4.14, -4.2, -4.26, -4.32, -4.38, -4.44, -4.5, 6.72, 6.66, 6.6000000000000005, 6.54, 6.48, 6.42, 6.36, 6.3, 6.24, 6.18, 6.12, 6.0600000000000005, 6.0, 5.94, -4.2, -4.26, -4.32, -4.38, -4.44, -4.5, -4.5600000000000005, -4.62, -4.68, -4.74, -4.8, -4.86, 7.2, 7.140000000000001, 7.08, 7.0200000000000005, 6.96, 6.9, 6.84, 6.78, 6.72, 6.66, 6.6000000000000005, 6.54, 6.48, 6.42, 6.36, 6.3, -4.44, -4.5, -4.5600000000000005, -4.62, -4.68, -4.74, -4.8, -4.86, -4.92, -4.98, -5.04, 7.5600000000000005, 7.5, 7.44, 7.38, 7.32, 7.26, 7.2, 7.140000000000001, 7.08, 7.0200000000000005, 6.96, 6.9, 6.84, 6.78, 6.72, 6.66, 6.6000000000000005, -4.74, -4.8, -4.86, -4.92, -4.98, -5.04, -5.1000000000000005, -5.16, -5.22, -5.28, 7.86, 7.8, 7.74, 7.68, 7.62, 7.5600000000000005, 7.5, 7.44, 7.38, 7.32, 7.26, 7.2, 7.140000000000001, 7.08, 7.0200000000000005, -4.98, -5.04, -5.1000000000000005, -5.16, -5.22, -5.28, -5.34, -5.4, -5.46, 7.98, 7.92, 7.86, 7.8, 7.74, 7.68, 7.62, 7.5600000000000005, 7.5, -5.04, -5.1000000000000005, -5.16, -5.22, -5.28, -5.34, -5.4, -5.46, -5.5200000000000005, -5.58, -5.64, -5.7, -5.76, 8.46, 8.4, 8.34, 8.28, 8.22, 8.16, 8.1, 8.040000000000001, 7.98, 7.92, 7.86, 7.8, 7.74, 7.68, 7.62, -5.22, -5.28, -5.34, -5.4, -5.46, -5.5200000000000005, -5.58, -5.64, -5.7, -5.76, -5.82, -5.88, -5.94, -6.0, -6.0600000000000005, -6.12, -6.18, -6.24, -6.3, 8.88, 8.82, 8.76, 8.700000000000001, 8.64, 8.58, 8.52, 8.46, 8.4, 8.34, 8.28, 8.22, 8.16, -5.64, -5.7, -5.76, -5.82, -5.88, -5.94, -6.0, -6.0600000000000005, -6.12, -6.18, -6.24, -6.3, -6.36, -6.42, 8.88, 8.82, 8.76, 8.52, 8.46, -6.0600000000000005, -6.12, -6.18, -6.24, -6.3, -6.36, -6.42, -5.16, -5.22, -5.28, -5.34, -5.4, -5.46, -5.5200000000000005, -5.58, -5.64, -4.92, -4.98, -5.04, -5.1000000000000005, -5.16, -5.22, -5.28, -5.34, -5.4, -5.46, -5.5200000000000005, -5.58, -5.64, -4.68, -4.74, -4.8, -4.86, -4.92, -4.98, -5.04, -5.1000000000000005, -5.16, -5.22, -5.28, -5.34, -5.4, -5.46, -4.32, -4.38, -4.44, -4.5, -4.5600000000000005, -4.62, -4.68, -4.74, -4.8, -4.0200000000000005, -4.08, -4.14, -4.2, -4.26, -4.32, -4.38, -4.44, -4.5, -4.5600000000000005, -4.62, -4.68, -3.84, -3.9, -3.96, -4.0200000000000005, -4.08, -4.14, -4.2, -4.26, -4.32, -4.38, -4.44, -4.5, 9.0, 8.94, 8.88, 8.82, 8.76, 8.700000000000001, 8.64, 8.58, 8.52, 8.46, -3.54, -3.6, -3.66, -3.72, -3.7800000000000002, -3.84, -3.9, -3.96, -4.0200000000000005, -4.08, 9.0, 8.94, 8.88, 8.82, 8.76, 8.700000000000001, 8.64, 8.58, 8.52, 8.46, 7.92, 7.86, 7.8, 7.74, 7.68, 7.62, 7.5600000000000005, 7.5, -3.3000000000000003, -3.36, -3.42, -3.48, -3.54, -3.6, -3.66, -3.72, -3.7800000000000002, -3.84, 7.92, 7.86, 7.8, 7.74, 7.68, 7.62, 7.5600000000000005, 7.5, 7.44, 7.38, 7.32, 7.26, 7.2, 7.140000000000001, 7.08, 7.0200000000000005, 6.96, 6.9, 6.84, 6.78, -2.94, -3.0, -3.06, -3.12, -3.18, -3.24, -3.3000000000000003, -3.36, -3.42, -3.48, -3.54, -3.6, 7.74, 7.68, 7.62, 7.5600000000000005, 7.5, 7.44, 7.38, 7.32, 7.26, 7.2, 7.140000000000001, 7.08, 7.0200000000000005, 6.96, 6.9, 6.84, 6.78, 6.72, 6.66, 6.6000000000000005, 6.54, 6.48, 6.42, -2.64, -2.7, -2.7600000000000002, -2.82, -2.88, -2.94, -3.0, -3.06, -3.12, -3.18, -3.24, -3.3000000000000003, -3.36, 7.26, 7.2, 7.140000000000001, 7.08, 7.0200000000000005, 6.96, 6.9, 6.84, 6.78, 6.72, 6.66, 6.6000000000000005, 6.54, 6.48, 6.42, 6.36, 6.3, 6.24, 6.18, 6.12, 6.0600000000000005, 6.0, -2.22, -2.2800000000000002, -2.34, -2.4, -2.46, -2.52, -2.58, -2.64, -2.7, -2.7600000000000002, -2.82, -2.88, -2.94, -3.0, -3.06, 6.36, 6.3, 6.24, 6.18, 6.12, 6.0600000000000005, 6.0, 5.94, 5.88, 5.82, 5.76, 5.7, -1.68, -1.74, -1.8, -1.86, -1.92, -1.98, -2.04, -2.1, -2.16, -2.22, -2.2800000000000002, -2.34, -2.4, -2.46, -2.52, -2.58, -2.64, 6.0600000000000005, 6.0, 5.94, 5.88, 5.82, 5.76, 5.7, 5.64, 5.58, 5.5200000000000005, 5.46, 5.4, 5.34, 5.28, 5.22, 5.16, 5.1000000000000005, 5.04, 4.98, -1.44, -1.5, -1.56, -1.62, -1.68, -1.74, -1.8, -1.86, -1.92, -1.98, -2.04, -2.1, -2.16, -2.22, -2.2800000000000002, 5.64, 5.58, 5.5200000000000005, 5.46, 5.4, 5.34, 5.28, 5.22, 5.16, 5.1000000000000005, 5.04, 4.98, 4.92, 4.86, 4.8, 4.74, 4.68, 4.62, 4.5600000000000005, 4.5, 4.44, 4.38, 4.32, -1.3800000000000001, -1.44, -1.5, -1.56, -1.62, -1.68, -1.74, -1.8, -1.86, -6.0600000000000005, -6.12, -6.18, 5.34, 5.28, 5.22, 5.16, 5.1000000000000005, 5.04, 4.98, 4.92, 4.86, 4.8, 4.74, 4.68, 4.62, 4.5600000000000005, 4.5, 4.44, 4.38, 4.32, 4.26, 4.2, 4.14, 4.08, 4.0200000000000005, 3.96, -1.1400000000000001, -1.2, -1.26, -1.32, -1.3800000000000001, -1.44, -1.5, -6.0, -6.0600000000000005, -6.12, -6.18, 4.86, 4.8, 4.74, 4.68, 4.62, 4.5600000000000005, 4.5, 4.44, 4.38, 4.32, 4.26, 4.2, 4.14, 4.08, 4.0200000000000005, 3.96, 3.9, 3.84, 3.7800000000000002, 3.72, -0.42, -0.48, -0.54, -0.6, -0.66, -0.72, -0.78, -0.84, -0.9, -0.96, -1.02, -1.08, -1.1400000000000001, -1.2, -1.26, -1.32, -5.94, -6.0, -6.0600000000000005, -6.12, 4.2, 4.14, 4.08, 4.0200000000000005, 3.96, 3.9, 3.84, 3.7800000000000002, 3.72, 3.66, 3.6, 3.54, 3.48, 3.42, 3.36, 3.3000000000000003, 3.24, 3.18, 3.12, 3.06, 3.0, 2.94, 2.88, 2.82, 2.7600000000000002, 2.7, 2.64, 2.58, 0.78, 0.72, 0.66, 0.6, 0.54, 0.48, 0.42, 0.36, 0.3, 0.24, 0.18, 0.12, 0.06, -0.0, -0.06, -0.12, -0.18, -0.24, -0.3, -0.36, -0.42, -0.48, -0.54, -0.6, -0.66, -0.72, -0.78, -0.84, -0.9, -0.96, -1.02, -1.08, -1.1400000000000001, -5.94, -6.0, 3.9, 3.84, 3.7800000000000002, 3.72, 3.66, 3.6, 3.54, 3.48, 3.42, 3.36, 3.3000000000000003, 3.24, 3.18, 3.12, 3.06, 3.0, 2.94, 2.88, 2.82, 2.7600000000000002, 2.7, 2.64, 2.58, 2.52, 2.46, 2.4, 2.34, 2.2800000000000002, 2.22, 2.16, 2.1, 2.04, 1.98, 1.92, 1.86, 1.8, 1.74, 1.68, 1.62, 1.56, 1.5, 1.44, 1.3800000000000001, 1.32, 1.26, 1.2, 1.1400000000000001, 1.08, 1.02, 0.96, 0.9, 0.84, 0.78, 0.72, 0.66, 0.6, 0.54, 0.48, 0.42, 0.36, 0.3, 0.24, 0.18, 0.12, 0.06, -0.0, -0.06, -0.12, -0.18, -0.24, -0.3, -0.36, -0.42, -0.48, -0.54, -0.6, -0.66, -0.72, -0.78, -0.84, -0.9, -0.96, -5.7, -5.76, -5.82, 3.84, 3.7800000000000002, 3.72, 3.66, 3.6, 3.54, 3.48, 3.42, 3.36, 3.3000000000000003, 3.24, 3.18, 3.12, 3.06, 3.0, 2.94, 2.88, 2.82, 2.7600000000000002, 2.7, 2.64, 2.58, 2.52, 2.46, 2.4, 2.34, 2.2800000000000002, 2.22, 2.16, 2.1, 2.04, 1.98, 1.92, 1.86, 1.8, 1.74, 1.68, 1.62, 1.56, 1.5, 1.44, 1.3800000000000001, 1.32, 1.26, 1.2, 1.1400000000000001, 1.08, 1.02, 0.96, 0.9, 0.84, 0.78, 0.72, 0.66, 0.6, 0.54, 0.48, 0.42, 0.36, 0.3, 0.24, 0.18, 0.12, 0.06, -0.0, -0.06, -0.12, -0.18, -5.64, -5.7, -5.76, -5.82, 2.4, 2.34, 2.2800000000000002, 2.22, 2.16, 2.1, 2.04, 1.98, 1.92, 1.86, -5.5200000000000005, -5.58, -5.64, -5.7, -5.34, -5.4, -5.46, -5.5200000000000005, -5.58, -5.22, -5.28, -5.34, -5.4, -5.46, -5.5200000000000005, -5.16, -5.22, -5.28, -5.34, -5.04, -5.1000000000000005, -5.16, -5.22, -5.28, -4.92, -4.98, -5.04, -5.1000000000000005, -5.16, -5.22, -4.92, -4.98, -5.04, -5.1000000000000005, -5.16, -4.74, -4.8, -4.86, -4.92, -4.98, -4.74, -4.8, -4.86, -4.92, -4.62, -4.68, -4.74, -4.8, -4.5, -4.5600000000000005, -4.62, -4.68, -4.74, -6.36, -6.42, -4.44, -4.5, -4.5600000000000005, -4.62, -4.68, -5.58, -5.64, -5.7, -6.36, -6.42]}]
  in  "Make WPT":bool
  in  "mission auto":bool=TRUE
  # "Traffic Signal"
  # "Sign Detection"
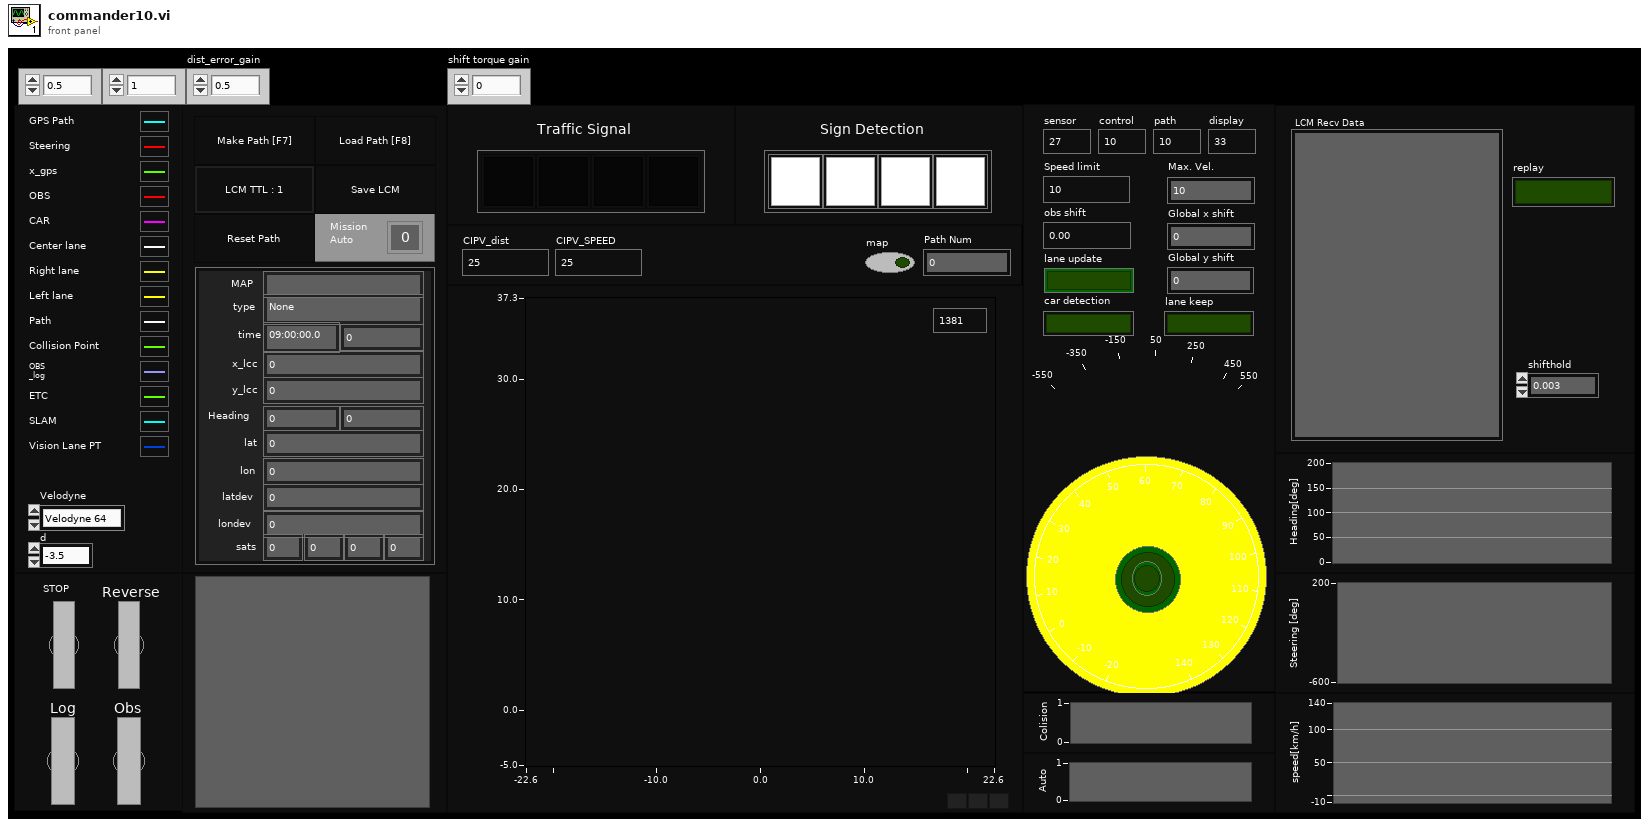
[diagram p1: front panel]
types:
  T1 = enum16{"Velodyne 16", "Velodyne 32", "Velodyne 64"}
  T2 = cluster{"type":string, "x_lcc":dbl, "y_lcc":dbl, "latdev":sgl, "londev":sgl, "sats":u8, "gps_l1_ranges":u8, "gps_l1_mask_ranges":u8, "gps_l2_mask_ranges":u8, "Heading":dbl, "lon":sgl, "lat":sgl, "time":string, "hgps":dbl, "lag":dbl, "MAP":string}
  T3 = cluster{"VS_des":dbl, "VS_can":dbl, "VS_des":dbl}
  T4 = enum8{"Enabled", "Disabled", "Disabled and Grayed Out"}
  T5 = typedef "Dynamixel Pro Driver.lvlib/Write Select Pro.ctl" = enum16{"ID", "Baud Rate", "Return Delay Time", "Operating mode", "Homing offset", "Moving threshold", "Temperature limit", "Max Voltage Limit", "Min Voltage Limit", "acceleration Limit", "Torque Limit", "Velocity Limit", "Max Position Limit", "Min Position Limit", "External Port Mode 1", "External Port Mode 2", "External Port Mode 3", "External Port Mode 4", "Shutdown", "Torque Enable", "LED RED", "LED GREEN", "LED BLUE", "Velocity I Gain", "Velocity P Gain", "Position P Gain", "Goal Position", "Goal Velocity", "Goal Torque", "Goal Acceleration", "External Port Data 1", "External Port Data 2", "External Port Data 3", "External Port Data 4", "Status Return Level"}
  T6 = typedef "Dynamixel Pro Driver.lvlib/Baudrate Selector.ctl" = enum16{"2400", "57600", "115200", "1000000", "2000000", "3000000", "4000000", "4500000", "10500000"}
  T7 = cluster{"Steer_input":dbl, "Steer_output":dbl, "VS_des":dbl, "VS_can":dbl, "heading":dbl, "auto":bool, "run":bool, "x":dbl, "y":dbl, "slam_y":dbl, "slam_x":dbl, "slam_heading":dbl}
  T8 = cluster{"hash":i64, "sys time":i64, "signal":i32, "sign":i32, "pedestrian":bool, "flag car":bool, "distance":dbl}
  T9 = typedef "imagedata.ctl" = cluster{"image type":i32, "image depth":i32, "image":u8[], "mask":u8[], "colors":u32[], "Rectangle":cluster{"left":i16, "top":i16, "right":i16, "bottom":i16}}
  T10 = cluster{"hash":i64, "sys time":i64, "status":i32, "TS_num":i32, "TS_type":i32[], "TS_loc_x":dbl[], "TS_loc_y":dbl[]}
  T11 = cluster{"hash":i64, "sys time":i64, "s_lat":dbl, "s_lon":dbl, "d_lat":dbl, "d_lon":dbl, "Message":i64}
  T12 = cluster{"beep":bool, "duration (msec)":u32, "frequency (Hz)":u32}
  T13 = enum32{"Namyang", "Hyundai", "KAIST", "Ajou", "Munji", "Airforce", "Car", "KATRI", "Samsung", "Coex", "Gwangnaru", "Inje", "sinjin", "NAVER"}
  T14 = cluster{"Minimum":dbl, "Minimum":dbl, "Minimum":dbl, "Minimum":dbl, "Minimum":dbl}
  T15 = cluster{"hash":i64, "sys time":i64, "time":dbl, "x":dbl, "y":dbl, "h":dbl, "numSV":i32, "postype":i32, "lag":i32, "hordev":dbl, "lat":dbl, "lon":dbl, "hgt":dbl, "map_idx":i32}
  T16 = cluster{"identifier":u32, "timestamp":timestamp, "payload":u8[]}
  T17 = cluster{"hash":i64, "sys time":i64, "size":i32, "data":u8[]}
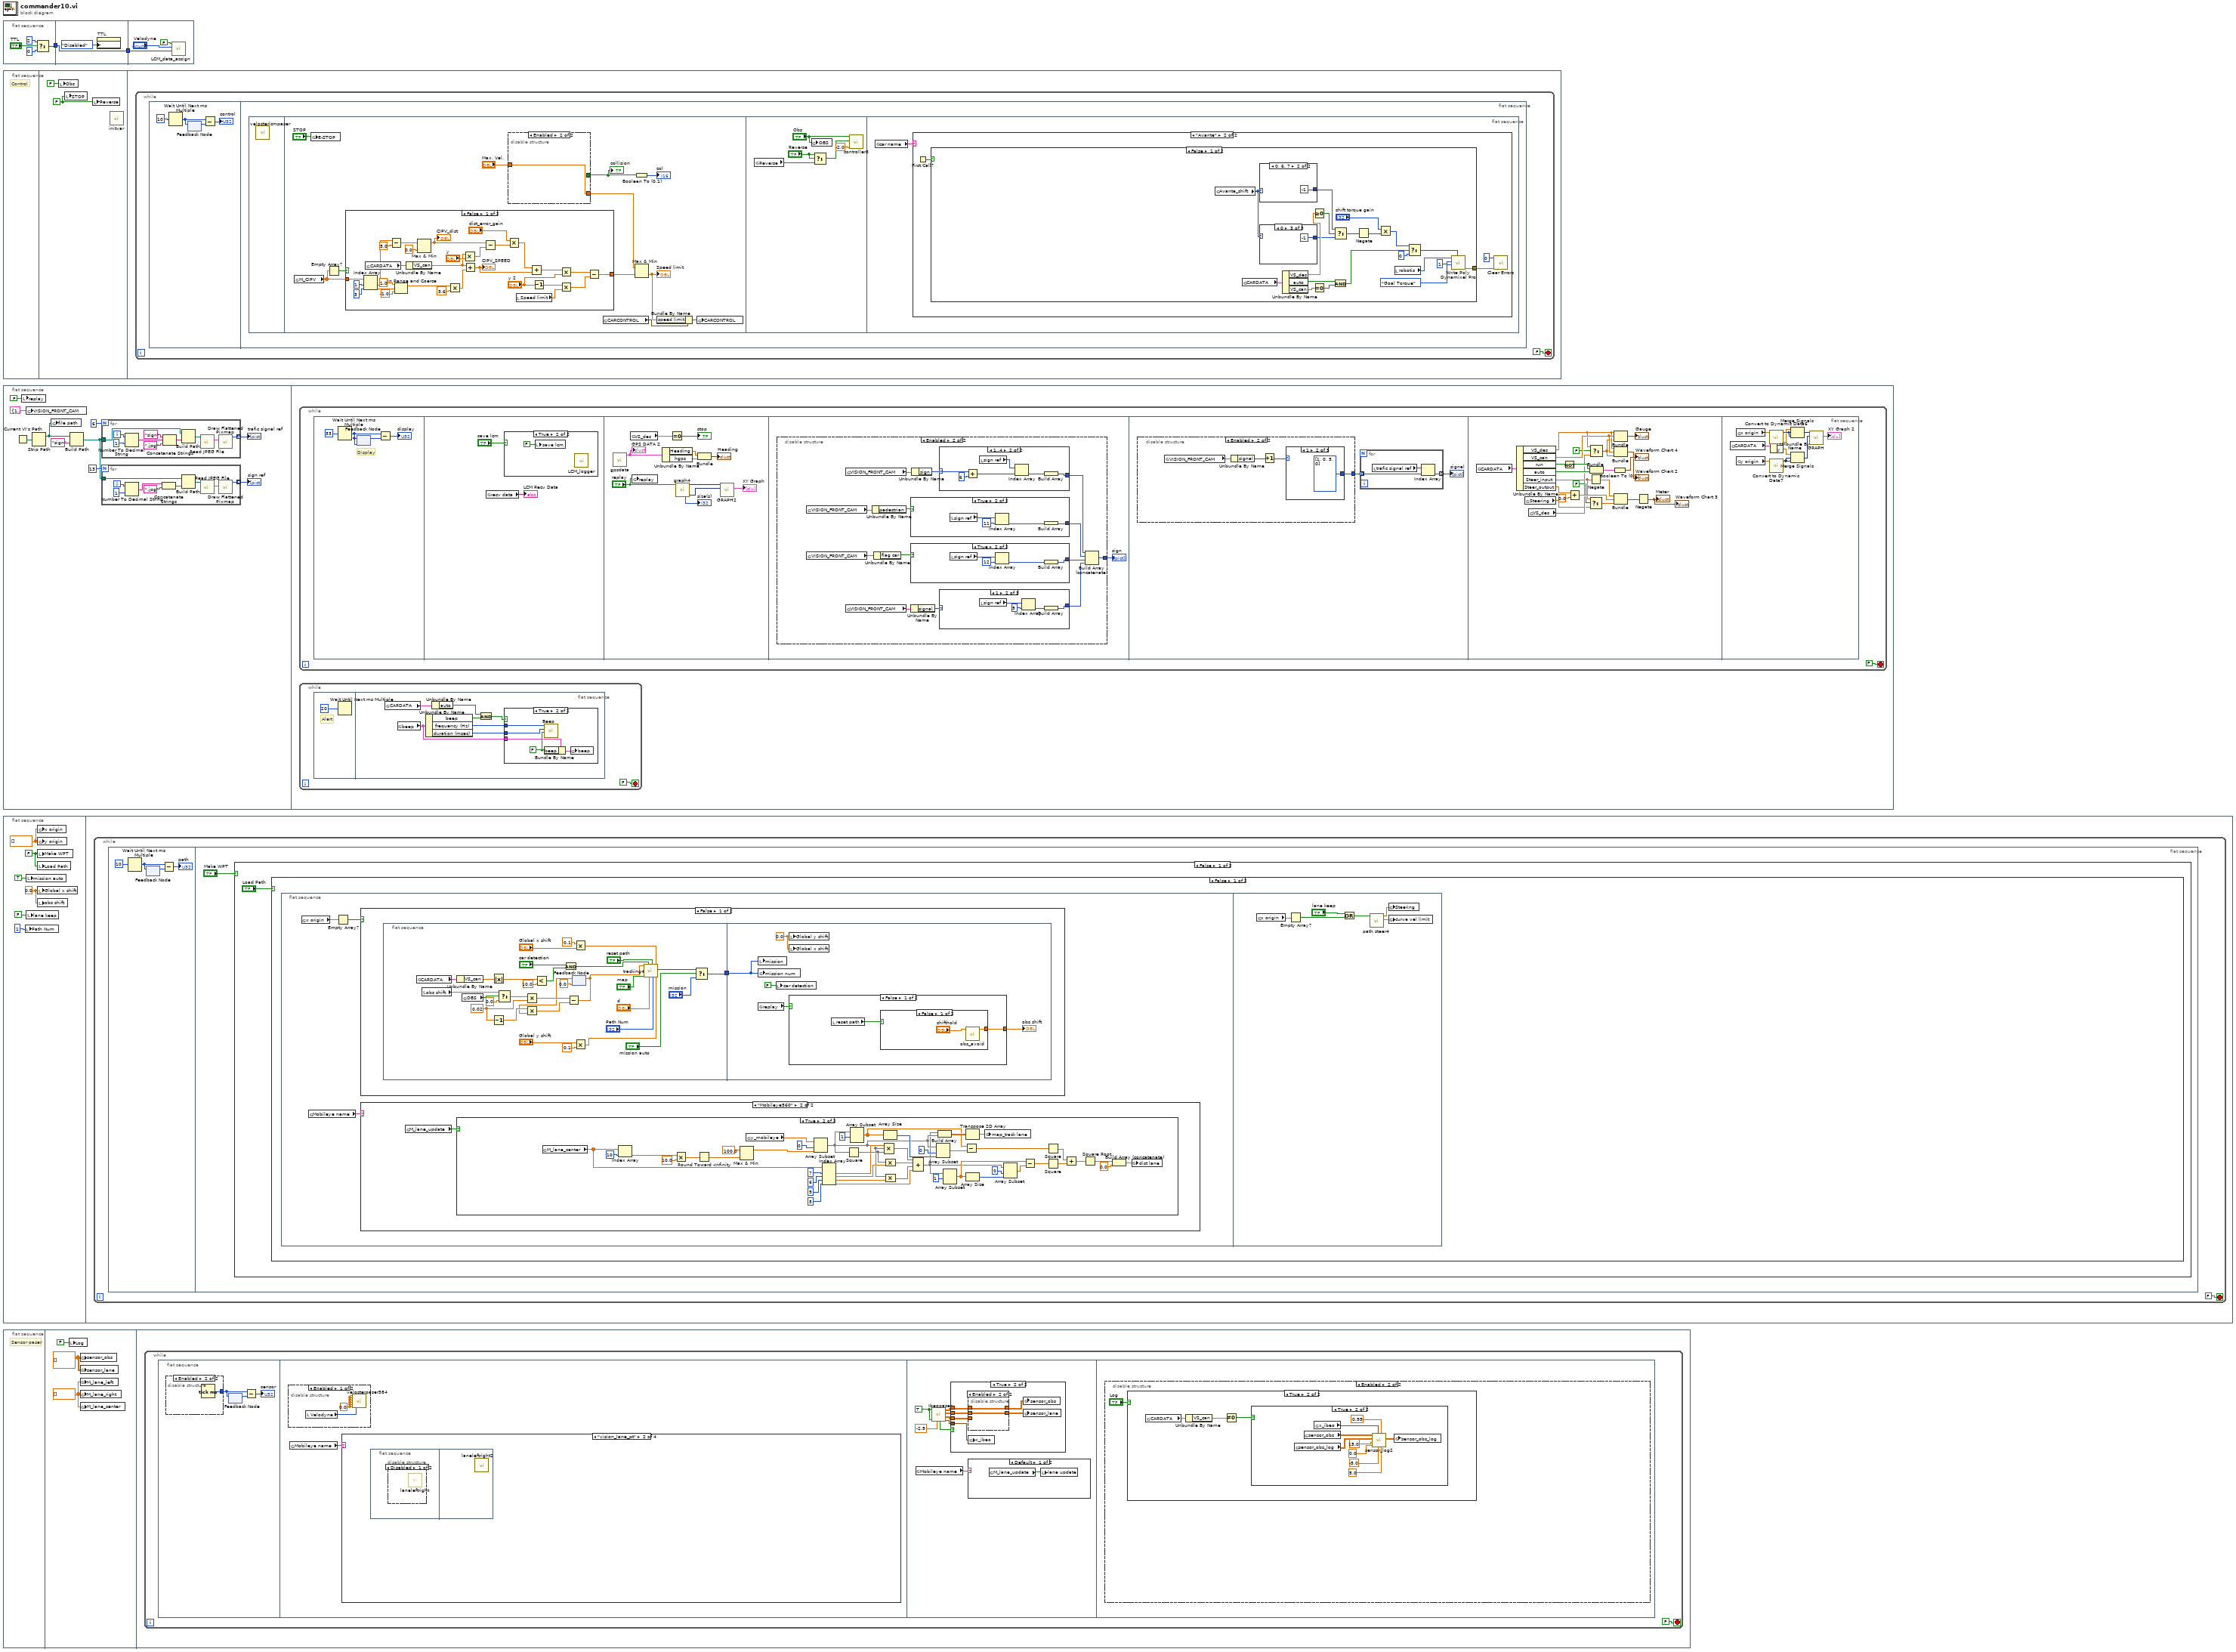
[diagram p0: block diagram]
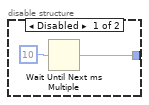
[diagram p2: hidden frame]
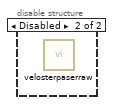
[diagram p3: hidden frame]
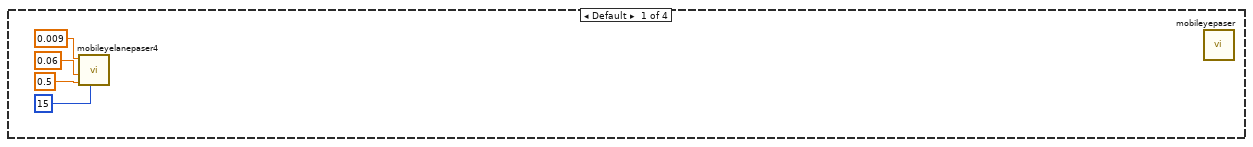
[diagram p4: hidden frame]
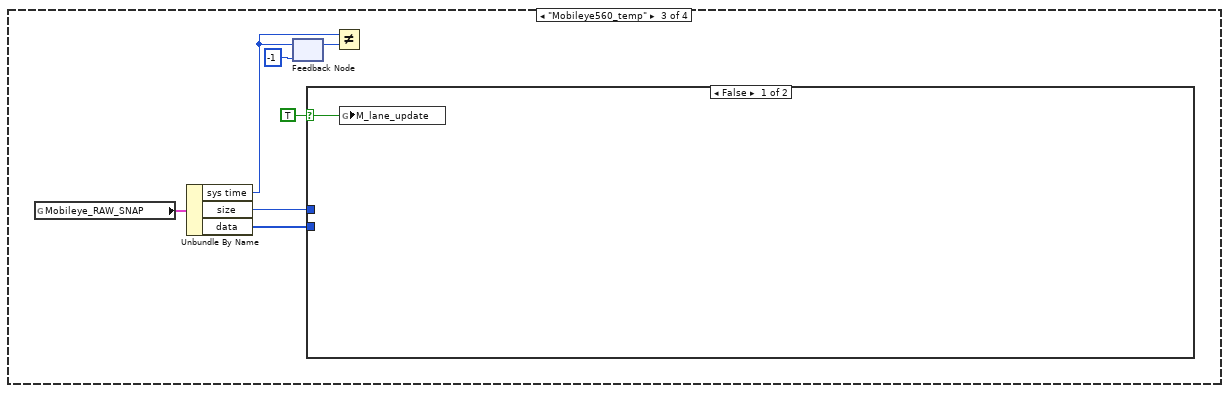
[diagram p6: hidden frame]
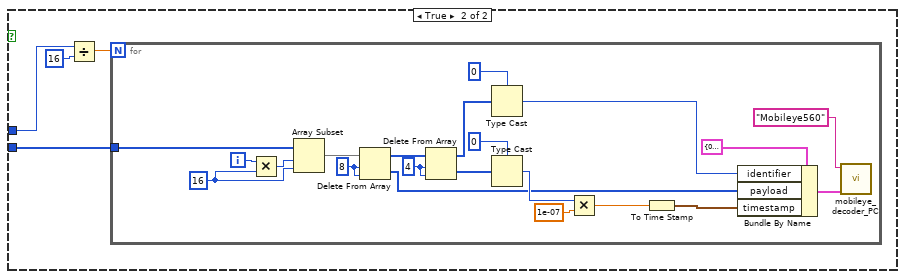
[diagram p7: hidden frame]
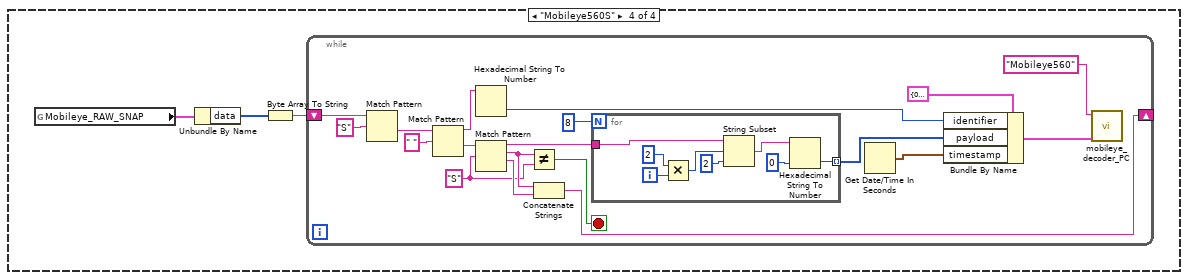
[diagram p8: hidden frame]
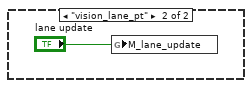
[diagram p9: hidden frame]
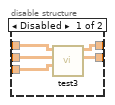
[diagram p11: hidden frame]
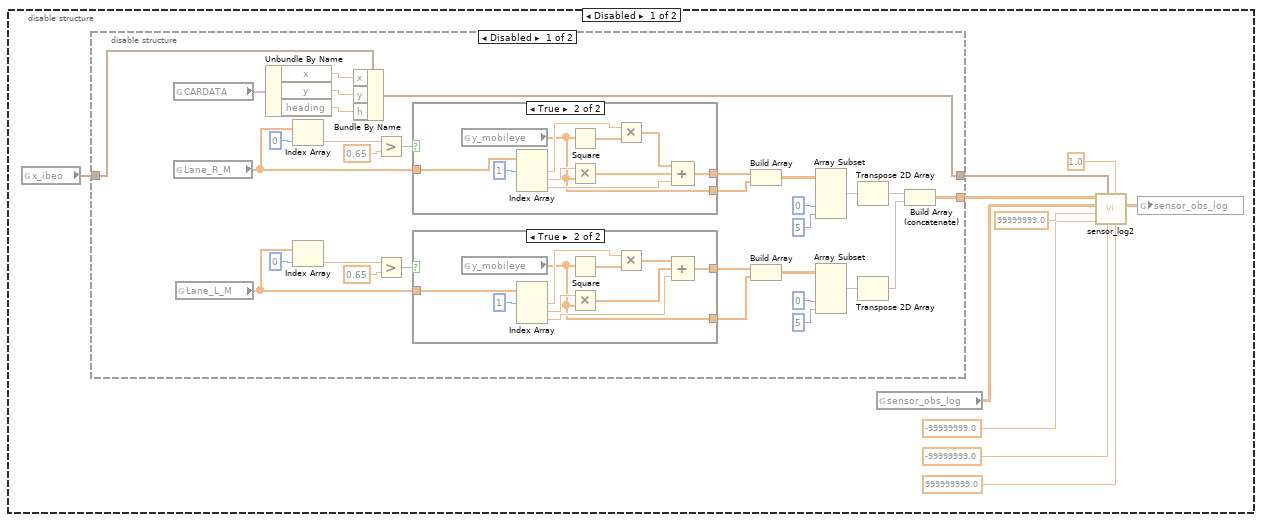
[diagram p12: hidden frame]
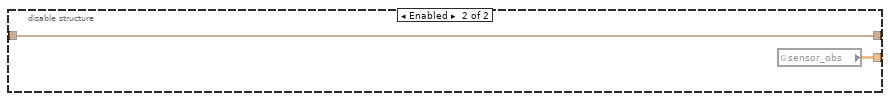
[diagram p15: hidden frame]
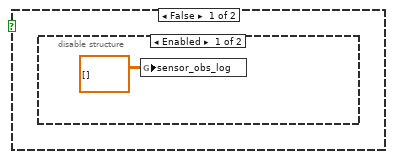
[diagram p16: hidden frame]
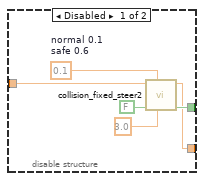
[diagram p19: hidden frame]
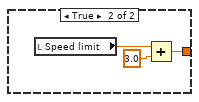
[diagram p20: hidden frame]
diagram:
  n1 = flat-sequence {
    tunnel: [w3] -> w1
    tunnel: [w7] -> w2
    tunnel: w1 -> [w7]
    tunnel: w2 -> [w9]
    frame #0 {
      n2 = Select(t=u16 2 ("time-to-live"), s="TTL", f=u16 0 ("time-to-live")) -> (s? t:f=w3:u16)
    }
    frame #1 {
      n3 = property on="TTL" class="Bool (strict)"("DisabledEnum"=T4."Disabled" ("Disabled")) -> ()  [unwired: 2 in, 2 out]
    }
    frame #2 {
      n4 = call "LCM_data_assign.vi"("time-to-live"=w9, "Velodyne1"="Velodyne", "velodyne enable"=FALSE) -> ()  [unwired: 9 in]
    }
  }
  n5 = flat-sequence {
    frame #0 {
      # "Control"
    }
    frame #1 {
      w13 = FALSE ("LCM")
      n6 = local write "Obs"(FALSE ("obs")) -> ()
      n7 = local write "STOP"(w13) -> ()
      n8 = local write "Reverse"(w13) -> ()
      n9 = call "initvar.vi"() -> ()  [unwired: 12 in]
    }
    frame #2 {
      n10 = while {
        stop <- FALSE ("Loop 1") stop-if-true
        n11 = flat-sequence {
          frame #0 {
            n12 = Wait Until Next ms Multiple(millisecond multiple=u32 10 ("milliseconds to wait")) -> (millisecond timer value=w15:u32)
            n13 = feedback #1() -> (w16:u32)  [unwired: 1 in]
            n14 = feedback-in #1(w15) -> ()
            n15 = Subtract(x=w15, y=w16) -> (x-y=→"control":u32)
          }
          frame #1 {
            n16 = flat-sequence {
              frame #0 {
                n17 = call "velosterlcmpaser.vi"() -> ()  [unwired: 11 in, 1 out]
              }
              frame #1 {
                n18 = global read "G_SEN.vi" "M_CIPV"() -> (w22:dbl[])
                n19 = global write "G_ALL.vi" "E-STOP"("STOP") -> ()
                n20 = Empty Array?(array=w22) -> (empty?=w23:bool)
                n21 = case shown="False" w23 {
                  tunnel: w22 -> [w65 _]
                  tunnel: [w48 w67] -> w19
                  frame False {
                    n22 = Index Array(array=w65, index #1=1 ("index"), index #2=3 ("index")) -> (element #1=w43:dbl, element #2=w47:dbl)
                    n23 = global read "G_ALL.vi" "CARDATA"() -> (w63:T7)
                    n24 = Subtract(x=w43, y=5.0) -> (x-y=w41:dbl)
                    n25 = In Range and Coerce(upper limit=1.0, x=w47, lower limit=-1.0) -> (coerced(x)=w44:dbl)  [unwired: 1 out]
                    n26 = Unbundle By Name(w63) -> ("VS_can"=w39:dbl)
                    n27 = Max & Min(x=w41, y=0.0) -> (max(x,y)=w38:dbl)  [unwired: 1 out]
                    "CIPV_dist" <- w38
                    n28 = Multiply(x=w44, y=3.6) -> (x*y=w57:dbl)
                    n29 = Multiply(x=w39, y="y") -> (x*y=w55:dbl)
                    n30 = Add(x=w39, y=w57) -> (x+y=w37:dbl)
                    "CIPV_SPEED" <- w37
                    n31 = Subtract(x=w38, y=w55) -> (x-y=w58:dbl)
                    n32 = Multiply(x="dist_error_gain", y=w58) -> (x*y=w60:dbl)
                    n33 = local read "Speed limit"() -> (w51:dbl)
                    n34 = Add(x=w60, y=w37) -> (x+y=w54:dbl)
                    n35 = Decrement(x="y 2") -> (x-1=w52:dbl)
                    n36 = Multiply(x=w54, y="y 2") -> (x*y=w49:dbl)
                    n37 = Multiply(x=w52, y=w51) -> (x*y=w50:dbl)
                    n38 = Subtract(x=w49, y=w50) -> (x-y=w48:dbl)
                  }
                  frame True {
                    n39 = local read "Speed limit"() -> (w68:dbl)
                    n40 = Add(x=w68, y=3.0) -> (x+y=w67:dbl)
                  }
                }
                n41 = disable-structure shown="Enabled" {
                  disable-tunnel: "Max. Vel." -> [w35 w36]
                  disable-tunnel: [w31 _] -> w27
                  disable-tunnel: [w30 w36] -> w21
                  frame Disabled {
                    w32 = 0.1  # normal 0.1 safe 0.6
                    n42 = call "collision_fixed_steer2.vi"("safe  dist"=3.0, "y"=w32, "obsclose"=FALSE, "Max. Vel."=w35) -> ("collision"=w31:bool, "speed limit"=w30:dbl)  [unwired: 5 in, 1 out]
                  }
                  frame Enabled {
                  }
                }
                "collision" <- w27
                n43 = global read "G_ALL.vi" "CARCONTROL"() -> (w25:cluster{"speed path":dbl, "speed limit":dbl})
                n44 = Boolean To (0,1)(Boolean=w27) -> (0, 1=→"col":i16)
                n45 = Max & Min(x=w21, y=w19) -> (min(x,y)=w20:dbl)  [unwired: 1 out]
                "Speed limit" <- w20
                n46 = Bundle By Name(cluster=w25, "speed limit"=w20) -> (w24:cluster{"speed path":dbl, "speed limit":dbl})
                n47 = global write "G_ALL.vi" "CARCONTROL"(w24) -> ()
              }
              frame #2 {
                n48 = global read "G_ALL.vi" "Reverse"() -> (w70:bool)
                n49 = global write "G_ALL.vi" "OBS"("Obs") -> ()
                n50 = Select(t="Reverse", s="Reverse", f=w70) -> (s? t:f=w72:bool)
                n51 = call "controller8.vi"("Neg max speed"=-2.0, "reverse"=w72, "obs"="Obs") -> ()  [unwired: 9 in]
              }
              frame #3 {
                n52 = global read "G_LCM.vi" "car name"() -> (w74:string)
                n53 = case shown="\"Avante\"" w74 {
                  frame Default {
                  }
                  frame "Avante" {
                    n54 = First Call?() -> (First Call?: T/F=w77:bool)
                    n55 = case shown="False" w77 {
                      tunnel: [w97 w103] -> w76
                      frame False {
                        n56 = global read "G_ALL.vi" "Avante_shift"() -> (w85:u8)
                        n57 = global read "G_ALL.vi" "CARDATA"() -> (w90:T7)
                        n58 = case shown="0, 6, 7" w85 {
                          tunnel: [0 -1] -> w83
                          frame 5, Default {
                          }
                          frame 0, 6, 7 {
                          }
                        }
                        n59 = case shown="0" w85 {
                          tunnel: [0 1 -1] -> w82
                          frame 7, Default {
                          }
                          frame 5, 6 {
                          }
                          frame 0 {
                          }
                        }
                        n60 = Unbundle By Name(w90) -> ("VS_des"=w86:dbl, "auto"=w88:bool, "VS_can"=w89:dbl)
                        n61 = Greater Or Equal To 0?(x=w86) -> (x >= 0?=w84:bool)
                        n62 = Equal To 0?(x=w89) -> (x = 0?=w87:bool)
                        n63 = And(x=w88, y=w87) -> (x .and. y?=w96:bool)
                        n64 = Select(t=w83, s=w84, f=w82) -> (s? t:f=w81:i32)
                        n65 = Negate(x=w81) -> (-x=w80:i32)
                        n66 = Multiply(x="shift torque gain", y=w80) -> (x*y=w92:i32)
                        n67 = local read "robotis"() -> (w79:refnum<visa-resource-name>)
                        n68 = Select(t=w92, s=w96, f=0) -> (s? t:f=w93:i32)
                        n69 = call-poly <vilib>:"Write Poly Dynamixel Pro.vi"("Value"=w93, "Operation"=Write_Select_Pro."Goal Torque", "ID"=u8 1, "VISA Refnum in"=w79) -> ("error out"=w97:errorcluster)  [unwired: 6 in, 1 out]
                      }
                      frame True {
                        n70 = flat-sequence {
                          tunnel: [w114] -> w111
                          tunnel: [w113] -> w110
                          tunnel: [w121] -> w109
                          tunnel: w111 -> [w121]
                          tunnel: [w120] -> w108
                          tunnel: w110 -> [w120]
                          tunnel: [w125] -> w107
                          tunnel: w109 -> [w127]
                          tunnel: w108 -> [w126]
                          tunnel: [w124] -> w106
                          tunnel: w107 -> [w131]
                          tunnel: [w131] -> w105
                          tunnel: [w130] -> w104
                          tunnel: w106 -> [w130]
                          tunnel: [w134] -> w103
                          tunnel: w105 -> [w136]
                          tunnel: w104 -> [w135]
                          frame #0 {
                            n71 = call <vilib>:"Open Session.vi"("Baud Rate"=Baudrate_Selector."57600", "VISA resource name"=refnum<visa-resource-name> "COM5") -> ("error out"=w117:errorcluster, "VISA Refnum out"=w118:refnum<visa-resource-name>)  [unwired: 8 in]
                            n72 = call-poly <vilib>:"Torque Poly.vi"("error in (no error)"=w117, "ID"=u8 1, "VISA Refnum in"=w118) -> ("error out"=w113:errorcluster, "VISA Refnum out"=w114:refnum<visa-resource-name>)  [unwired: 7 in]
                          }
                          frame #1 {
                            n73 = Wait (ms)(milliseconds to wait=u32 2000) -> ()  [unwired: 1 out]
                          }
                          frame #2 {
                            n74 = call-poly <vilib>:"Write Poly Dynamixel Pro.vi"("Value"=0, "error in (no error)"=w126, "Operation"=Write_Select_Pro."Operating mode", "ID"=u8 1, "VISA Refnum in"=w127) -> ("error out"=w124:errorcluster, "VISA Refnum out"=w125:refnum<visa-resource-name>)  [unwired: 5 in]
                          }
                          frame #3 {
                            n75 = Wait (ms)(milliseconds to wait=u32 2000) -> ()  [unwired: 1 out]
                          }
                          frame #4 {
                            n76 = call-poly <vilib>:"Torque Poly.vi"("error in (no error)"=w135, "ID"=u8 1, "VISA Refnum in"=w136) -> ("error out"=w134:errorcluster, "VISA Refnum out"=→"robotis":refnum<visa-resource-name>)  [unwired: 7 in]
                          }
                        }
                      }
                    }
                    n77 = call <vilib>:"Clear Errors.vi"("error in (no error)"=w76, "specific error code to clear (0: all)"=0) -> ()  [unwired: 4 in, 2 out]
                  }
                }
              }
            }
          }
        }
      }
    }
  }
  n78 = flat-sequence {
    frame #0 {
      n79 = Current VI's Path() -> (path=w145:path)
      n80 = local write "replay"(FALSE ("replay")) -> ()
      n81 = global write "G_LCM.vi" "VISION_FRONT_CAM"(T8 {"hash"=1386151893206175709, "sys time"=1, "signal"=1, "sign"=3, "pedestrian"=TRUE, "flag car"=TRUE, "distance"=0.0} ("VISION_FRONT_CAM")) -> ()
      n82 = Strip Path(path=w145) -> (stripped path=w138:path)  [unwired: 1 out]
      n83 = global write "G_ALL.vi" "file path"(w138) -> ()
      n84 = Build Path(base path=w138, name or relative path="sign") -> (appended path=w139:path)
      n85 = for {
        N: 6 -> [_]
        tunnel: [w155] -> w141 mode=indexing
        tunnel: w139 -> [w150]
        i -> [w154]
        n86 = Number To Decimal String(number=w154, width (-)=i16 1) -> (decimal integer string=w152:string)
        n87 = Concatenate Strings("sign" ("string"), w152, ".jpg") -> (w149:string)
        n88 = Build Path(base path=w150, name or relative path=w149) -> (appended path=w148:path)
        n89 = call <vilib>:"Read JPEG File.vi"("path to JPEG file"=w148) -> ("image data"=w156:T9)  [unwired: 8 in, 2 out]
        n90 = call <vilib>:"Draw Flattened Pixmap.vi"("image data"=w156) -> ("new picture"=w155:picture)  [unwired: 8 in]
      }
      "trafic signal ref" <- w141
      n91 = for {
        N: 13 -> [_]
        tunnel: [w164] -> w142 mode=indexing
        tunnel: w139 -> [w159]
        i -> [w163]
        n92 = Number To Decimal String(number=w163, width (-)=i16 1) -> (decimal integer string=w161:string)
        n93 = Concatenate Strings(w161, ".jpg") -> (w158:string)
        n94 = Build Path(base path=w159, name or relative path=w158) -> (appended path=w157:path)
        n95 = call <vilib>:"Read JPEG File.vi"("path to JPEG file"=w157) -> ("image data"=w165:T9)  [unwired: 8 in, 2 out]
        n96 = call <vilib>:"Draw Flattened Pixmap.vi"("image data"=w165) -> ("new picture"=w164:picture)  [unwired: 8 in]
      }
      "sign ref" <- w142
    }
    frame #1 {
      n97 = while {
        stop <- FALSE ("Loop 2") stop-if-true
        n98 = flat-sequence {
          frame #0 {
            # "Display"
            n99 = Wait Until Next ms Multiple(millisecond multiple=u32 33 ("milliseconds to wait")) -> (millisecond timer value=w181:u32)
            n100 = feedback #2(w181) -> (w183:u32)
            n101 = feedback-in #2(w181) -> ()
            n102 = Subtract(x=w181, y=w183) -> (x-y=→"display":u32)
          }
          frame #1 {
            n103 = global read "G_LCM.vi" "recv data"() -> (→"LCM Recv Data":string)
            n104 = case shown="True" "save lcm" {
              frame False {
              }
              frame True {
                n105 = local write "save lcm"(FALSE ("save lcm")) -> ()
                n106 = call "LCM_logger.vi"() -> ()  [unwired: 12 in]
              }
            }
          }
          frame #2 {
            n107 = call "gpsdata.vi"() -> ("GPS DATA 2"=w191:T2)  [unwired: 11 in]
            "GPS DATA 2" <- w191
            n108 = global read "G_ALL.vi" "VS_des"() -> (w197:dbl)
            n109 = global write "G_ALL.vi" "replay"("replay") -> ()
            n110 = Unbundle By Name(w191) -> ("Heading"=w189:dbl, "hgps"=w190:dbl)
            n111 = Equal To 0?(x=w197) -> (x = 0?=→"stop":bool)
            n112 = call "graph4.vi"("replay"="replay") -> ("y"=w195:dynamicdata, "x"=w194:dynamicdata, "size(s)"=→"size(s)":i32)  [unwired: 8 in]
            n113 = Bundle("Heading"=w189, "hgps"=w190) -> (→"Heading":cluster{"Heading":dbl, "hgps":dbl})  [unwired: 1 in]
            n114 = call "GRAPH2"("Y Input"=w195, "X Input"=w194) -> ("XY Graph"=→"XY Graph":cluster{"Y":dbl[], "Y":dbl[]}[])  [unwired: 3 in, 6 out]
          }
          frame #3 {
            n115 = disable-structure shown="Enabled" {
              disable-tunnel: [w202 w225] -> w199
              frame Disabled {
                n116 = global read "G_LCM.vi" "EURECAR_VISION"() -> (w203:T10)
                n117 = Unbundle By Name(w203) -> ("TS_num"=w200:i32, "TS_type"=w201:i32[])
                n118 = case shown="0" w200 {
                  tunnel: w201 -> [_ w214]
                  tunnel: [w208 w213] -> w202
                  frame 0 {
                    w210 = 100 ("x")
                    n119 = local read "count"() -> (w211:i32)
                    n120 = Increment(x=w211) -> (x+1=w206:i32)
                    n121 = Max & Min(x=w210, y=w206) -> (min(x,y)=w205:i32)  [unwired: 1 out]
                    n122 = local write "count"(w205) -> ()
                    n123 = Equal?(x=w210, y=w205) -> (x = y?=w204:bool)
                    n124 = local read "sign"() -> (w207:picture[])
                    n125 = Select(t=picture[] [], s=w204, f=w207) -> (s? t:f=w208:picture[])
                  }
                  frame 1, Default {
                    n126 = for {
                      tunnel: w214 -> [w216] mode=indexing
                      tunnel: [w215] -> w213 mode=indexing
                      n127 = local read "sign ref"() -> (w217:picture[])
                      n128 = Index Array(array=w217, index=w216) -> (element=w215:picture)
                    }
                    "count" <- 0 ("Numeric Control")
                  }
                }
              }
              frame Enabled {
                n129 = global read "G_LCM.vi" "VISION_FRONT_CAM"() -> (w224:T8)
                n130 = global read "G_LCM.vi" "VISION_FRONT_CAM"() -> (w223:T8)
                n131 = global read "G_LCM.vi" "VISION_FRONT_CAM"() -> (w229:T8)
                n132 = global read "G_LCM.vi" "VISION_FRONT_CAM"() -> (w220:T8)
                n133 = Unbundle By Name(w224) -> ("pedestrian"=w228:bool)
                n134 = Unbundle By Name(w223) -> ("flag car"=w222:bool)
                n135 = case shown="True" w228 {
                  tunnel: [picture[] [] w246] -> w227
                  frame False {
                  }
                  frame True {
                    n136 = local read "sign ref"() -> (w249:picture[])
                    n137 = Index Array(array=w249, index=11) -> (element=w247:picture)
                    n138 = Build Array(w247) -> (w246:picture[])
                  }
                }
                n139 = case shown="True" w222 {
                  tunnel: [picture[] [] w241] -> w221
                  frame False {
                  }
                  frame True {
                    n140 = local read "sign ref"() -> (w244:picture[])
                    n141 = Index Array(array=w244, index=12) -> (element=w242:picture)
                    n142 = Build Array(w242) -> (w241:picture[])
                  }
                }
                n143 = Unbundle By Name(w220) -> ("signal"=w219:i32)
                n144 = Unbundle By Name(w229) -> ("sign"=w230:i32)
                n145 = case shown="1..4" w230 {
                  selector: w230 -> [_ w255]
                  tunnel: [picture[] [] w251] -> w226
                  frame 0, Default {
                  }
                  frame 1..4 {
                    n146 = Add(x=w255, y=6) -> (x+y=w253:i32)
                    n147 = local read "sign ref"() -> (w256:picture[])
                    n148 = Index Array(array=w256, index=w253) -> (element=w252:picture)
                    n149 = Build Array(w252) -> (w251:picture[])
                  }
                }
                n150 = case shown="1" w219 {
                  selector: w219 -> [_ _ w238]
                  tunnel: [picture[] [] w233 w236] -> w218
                  frame 0, Default {
                  }
                  frame 1 {
                    n151 = local read "sign ref"() -> (w235:picture[])
                    n152 = Index Array(array=w235, index=5) -> (element=w234:picture)
                    n153 = Build Array(w234) -> (w233:picture[])
                  }
                  frame 5 {
                    n154 = local read "sign ref"() -> (w239:picture[])
                    n155 = Index Array(array=w239, index=w238) -> (element=w237:picture)
                    n156 = Build Array(w237) -> (w236:picture[])
                  }
                }
                n157 = Build Array (concatenate)(w226, w227, w221, w218) -> (w225:picture[])
              }
            }
            "sign" <- w199
          }
          frame #4 {
            n158 = disable-structure shown="Enabled" {
              disable-tunnel: [w265 w274] -> w258
              frame Disabled {
                n159 = global read "G_LCM.vi" "APP_GPS_DATA"() -> (w264:T11)
                n160 = Unbundle By Name(w264) -> ("Message"=w263:i64)
                n161 = case shown="1" w263 {
                  tunnel: [_ TRUE _ _] -> _
                  tunnel: [i32[] [0, 5, 0, 0] i32[] [1, 5, 0, 0] i32[] [0, 2, 0, 0] i32[] [0, 5, 3, 0]] -> w265
                  frame 0, Default {
                  }
                  frame 1 {
                  }
                  frame 2 {
                  }
                  frame 3 {
                  }
                }
                n162 = Equal To 0?(x=w263) -> (x = 0?=w262:bool)
                n163 = Select(t="", s=w262, f="미션중") -> (s? t:f=w259:string)
              }
              frame Enabled {
                n164 = global read "G_LCM.vi" "VISION_FRONT_CAM"() -> (w273:T8)
                n165 = Unbundle By Name(w273) -> ("signal"=w272:i32)
                n166 = Increment(x=w272) -> (x+1=w271:i32)
                n167 = case shown="1" w271 {
                  tunnel: [i32[] [0, 0, 5, 0] i32[] [1, 0, 5, 0] i32[] [0, 4, 5, 0] i32[] [0, 0, 2, 0] i32[] [0, 0, 5, 3]] -> w274
                  frame 0, Default {
                  }
                  frame 1 {
                  }
                  frame 2 {
                  }
                  frame 3 {
                  }
                  frame 4 {
                  }
                }
              }
            }
            n168 = for {
              tunnel: w258 -> [w281] mode=indexing
              tunnel: [w280] -> w257 mode=indexing
              n169 = local read "trafic signal ref"() -> (w282:picture[])
              n170 = Index Array(array=w282, index=w281) -> (element=w280:picture)
            }
            "signal" <- w257
          }
          frame #5 {
            n171 = global read "G_ALL.vi" "CARDATA"() -> (w289:T7)
            n172 = Unbundle By Name(w289) -> ("VS_des"=w292:dbl, "VS_can"=w299:dbl, "run"=w297:bool, "auto"=w298:bool, "Steer_input"=w284:dbl, "Steer_output"=w296:dbl)
            n173 = global read "G_ALL.vi" "Steering"() -> (w285:dbl)
            n174 = global read "G_ALL.vi" "VS_des"() -> (w288:dbl)
            n175 = Not(x=w297) -> (.not. x?=w301:bool)
            n176 = Add(x=w296, y=0.0) -> (x+y=w294:dbl)
            n177 = Negate(x=w284) -> (-x=w283:dbl)
            n178 = Select(t=w284, s=FALSE, f=w285) -> (s? t:f=w293:dbl)
            n179 = Select(t=w292, s=FALSE, f=w288) -> (s? t:f=w291:dbl)
            n180 = Bundle(w301, "auto"=w298) -> (w303:cluster{bool, "auto":bool})  [unwired: 1 in]
            n181 = Boolean To (0,1)(Boolean=w303) -> (0, 1=→"Waveform Chart 4":cluster{i16, "auto":i16})
            n182 = Bundle("VS_des"=w292, "VS_can"=w299, "VS_des"=w291) -> (→"Gauge":T3)  [unwired: 1 in]
            n183 = Bundle("VS_des"=w292, "VS_can"=w299, "VS_des"=w291) -> (→"Waveform Chart 2":T3)  [unwired: 1 in]
            n184 = Bundle(w283, w294, "Steering"=w293) -> (w305:cluster{dbl, dbl, "Steering":dbl})  [unwired: 1 in]
            n185 = Negate(x=w305) -> (-x=→"Meter" →"Waveform Chart 3":cluster{dbl, dbl, "Steering":dbl})
          }
          frame #6 {
            n186 = global read "G_ALL.vi" "CARDATA"() -> (w308:T7)
            n187 = global read "G_ALL.vi" "x origin"() -> (w307:dbl[])
            n188 = global read "G_ALL.vi" "y origin"() -> (w306:dbl[])
            n189 = call "Convert to Dynamic Data6"("Array"=w307) -> ("Dynamic Data Type"=w315:dynamicdata)  [unwired: 3 in]
            n190 = call "Convert to Dynamic Data7"("Array"=w306) -> ("Dynamic Data Type"=w314:dynamicdata)  [unwired: 3 in]
            n191 = Unbundle By Name(w308) -> ("x"=w312:dbl, "y"=w313:dbl)
            n192 = Merge Signals(w312, w315, w315) -> (w310:dynamicdata)
            n193 = Merge Signals(w313, w314, w314) -> (w309:dynamicdata)
            n194 = call "GRAPH"("Y Input"=w309, "X Input"=w310) -> ("XY Graph"=→"XY Graph 2":cluster{"Y":dbl[], "Y":dbl[]}[])  [unwired: 3 in, 6 out]
          }
        }
      }
      n195 = while {
        stop <- FALSE stop-if-true
        n196 = flat-sequence {
          frame #0 {
            # "Alert"
            n197 = Wait Until Next ms Multiple(millisecond multiple=u32 20 ("millisecond timer value")) -> ()  [unwired: 1 out]
          }
          frame #1 {
            n198 = global read "G_ALL.vi" "CARDATA"() -> (w171:T7)
            n199 = global read "G_ALL.vi" "beep"() -> (w172:T12)
            n200 = Unbundle By Name(w172) -> ("beep"=w169:bool, "frequency (Hz)"=w174:u32, "duration (msec)"=w173:u32)
            n201 = Unbundle By Name(w171) -> ("auto"=w170:bool)
            n202 = And(x=w170, y=w169) -> (x .and. y?=w168:bool)
            n203 = case shown="True" w168 {
              tunnel: w174 -> [_ w179]
              tunnel: w173 -> [_ w178]
              tunnel: w172 -> [_ w175]
              frame False {
              }
              frame True {
                w177 = FALSE ("use system alert? (T)")
                n204 = call <vilib>:"Beep.vi"("use system alert? (T)"=w177, "duration (msec)"=w178, "frequency (Hz)"=w179) -> ()  [unwired: 9 in]
                n205 = Bundle By Name(cluster=w175, "beep"=w177) -> (w176:T12)
                n206 = global write "G_ALL.vi" "beep"(w176) -> ()
              }
            }
          }
        }
      }
    }
  }
  n207 = flat-sequence {
    frame #0 {
      w319 = dbl[] [] ("x origin")
      w320 = 0.0 ("x")
      w321 = FALSE ("Make WPT")
      n208 = local write "Path Num"(1 ("milliseconds to wait")) -> ()
      n209 = local write "mission auto"(TRUE ("mission auto")) -> ()
      n210 = local write "lane keep"(FALSE ("lane update")) -> ()
      n211 = global write "G_ALL.vi" "x origin"(w319) -> ()
      n212 = global write "G_ALL.vi" "y origin"(w319) -> ()
      n213 = local write "Make WPT"(w321) -> ()
      n214 = local write "Load Path"(w321) -> ()
      n215 = local write "Global x shift"(w320) -> ()
      n216 = local write "obs shift"(w320) -> ()
    }
    frame #1 {
      n217 = while {
        stop <- FALSE ("Loop 3") stop-if-true
        n218 = flat-sequence {
          frame #0 {
            n219 = Wait Until Next ms Multiple(millisecond multiple=u32 10 ("milliseconds to wait")) -> (millisecond timer value=w323:u32)
            n220 = feedback #3() -> (w325:u32)  [unwired: 1 in]
            n221 = feedback-in #3(w323) -> ()
            n222 = Subtract(x=w323, y=w325) -> (x-y=→"path":u32)
          }
          frame #1 {
            n223 = case shown="False" "Make WPT" {
              frame False {
                n224 = case shown="False" "Load Path" {
                  frame False {
                    n225 = flat-sequence {
                      frame #0 {
                        n226 = global read "G_ALL.vi" "x origin"() -> (w331:dbl[])
                        n227 = global read "G_LCM.vi" "Mobileye name"() -> (w329:string)
                        n228 = Empty Array?(array=w331) -> (empty?=w330:bool)
                        n229 = case shown="False" w330 {
                          frame False {
                            n230 = flat-sequence {
                              tunnel: [w380] -> w377
                              tunnel: w377 -> [w410]
                              frame #0 {
                                w407 = 0.02 ("y")
                                n231 = global read "G_ALL.vi" "CARDATA"() -> (w392:T7)
                                n232 = local read "obs shift"() -> (w409:dbl)
                                n233 = Unbundle By Name(w392) -> ("VS_can"=w391:dbl)
                                n234 = global read "G_ALL.vi" "OBS"() -> (w385:bool)
                                n235 = Absolute Value(x=w391) -> (abs(x)=w390:dbl)
                                n236 = Decrement(x=w407) -> (x-1=w405:dbl)
                                n237 = Select(t=w409, s=w385, f=0.0) -> (s? t:f=w399:dbl)
                                n238 = Multiply(x=w399, y=w407) -> (x*y=w406:dbl)
                                n239 = Less?(x=w390, y=10.0) -> (x < y?=w388:bool)
                                n240 = And(x="car detection", y=w388) -> (x .and. y?=w386:bool)
                                n241 = feedback #4(0.0) -> (w404:dbl)
                                n242 = Multiply(x=w405, y=w404) -> (x*y=w403:dbl)
                                n243 = Subtract(x=w406, y=w403) -> (x-y=w402:dbl)
                                n244 = feedback-in #4(w402) -> ()
                                n245 = Multiply(x=0.1 ("y"), y="Global x shift") -> (x*y=w397:dbl)
                                n246 = Multiply(x="Global y shift", y=0.1) -> (x*y=w395:dbl)
                                n247 = call "tracking4.vi"("y"=w395, "x"=w397, "path num"="Path Num", "reset path"="reset path", "d"="d", "car detection"=w386, "map"="map", "xt"=w402) -> ("mission"=w382:i32)  [unwired: 3 in]
                                n248 = Select(t=w382, s="mission auto", f="mission") -> (s? t:f=w380:i32)
                              }
                              frame #1 {
                                w413 = 0.0 ("x")
                                n249 = local write "mission"(w410) -> ()
                                n250 = global write "G_ALL.vi" "mission num"(w410) -> ()
                                n251 = global read "G_ALL.vi" "replay"() -> (w411:bool)
                                n252 = local write "car detection"(FALSE ("car detection")) -> ()
                                n253 = local write "Global y shift"(w413) -> ()
                                n254 = local write "Global x shift"(w413) -> ()
                                n255 = case shown="False" w411 {
                                tunnel: [w416 _] -> w412
                                frame False {
                                n256 = local read "reset path"() -> (w415:bool)
                                n257 = case shown="False" w415 {
                                tunnel: [w418 _] -> w416
                                frame False {
                                n258 = call "obs_avoid.vi"("shifthold"="shifthold") -> ("obs shift"=w418:dbl)  [unwired: 10 in]
                                }
                                frame True {
                                n259 = local write "reset path"(FALSE ("reset path")) -> ()
                                }
                                }
                                }
                                frame True {
                                }
                                }
                                "obs shift" <- w412
                              }
                            }
                          }
                          frame True {
                          }
                        }
                        n260 = case shown="\"Mobileye560\"" w329 {
                          frame Default {
                          }
                          frame "Mobileye560" {
                            n261 = global read "G_SEN.vi" "M_lane_update"() -> (w332:bool)
                            n262 = case shown="True" w332 {
                              frame False {
                              }
                              frame True {
                                n263 = global read "G_SEN.vi" "M_lane_center"() -> (w356:dbl[])
                                n264 = Index Array(array=w356, index=10) -> (element=w362:dbl)
                                n265 = Multiply(x=w362, y=10.0) -> (x*y=w373:dbl)
                                n266 = Round Toward -Infinity(1:w373) -> (0:w359:dbl)
                                n267 = Max & Min(x=100.0, y=w359) -> (max(x,y)=w376:dbl)  [unwired: 1 out]
                                n268 = global read "G_SEN.vi" "y_mobileye"() -> (w353:dbl[])
                                n269 = Array Subset(array=w353, index=0, length=w376) -> (w335:dbl[])
                                n270 = Index Array(array=w356, index #1=7 ("index"), index #2=6 ("index"), index #3=9 ("index"), index #4=5 ("index")) -> (element #1=w357:dbl, element #2=w370:dbl, element #3=w368:dbl, element #4=w375:dbl)
                                n271 = Square(x=w335) -> (x^2=w364:dbl[])
                                n272 = Array Subset(array=w335, index=1) -> (w347:dbl[])  [unwired: 1 in]
                                n273 = Array Size(array=w347) -> (size(s)=w344:i32)
                                n274 = Compound Arithmetic op=MULTIPLY(w357, w335, w364) -> (w367:dbl[])
                                n275 = Compound Arithmetic op=MULTIPLY(w364, w370) -> (w366:dbl[])
                                n276 = Compound Arithmetic op=MULTIPLY(w335, w368) -> (w365:dbl[])
                                n277 = Compound Arithmetic op=ADD(w367, w366, w365, w375) -> (w334:dbl[])
                                n278 = Array Subset(array=w335, index=0, length=w344) -> (w346:dbl[])
                                n279 = Build Array(w334, w335) -> (w354:dbl[][])
                                n280 = Array Subset(array=w334, index=1) -> (w348:dbl[])  [unwired: 1 in]
                                n281 = Subtract(x=w347, y=w346) -> (x-y=w342:dbl[])
                                n282 = Transpose 2D Array(2D array=w354) -> (transposed array=w355:dbl[][])
                                n283 = Array Size(array=w348) -> (size(s)=w351:i32)
                                n284 = global write "G_ALL.vi" "map_track lane"(w355) -> ()
                                n285 = Array Subset(array=w334, index=0, length=w351) -> (w349:dbl[])
                                n286 = Subtract(x=w348, y=w349) -> (x-y=w341:dbl[])
                                n287 = Square(x=w342) -> (x^2=w340:dbl[])
                                n288 = Square(x=w341) -> (x^2=w339:dbl[])
                                n289 = Add(x=w340, y=w339) -> (x+y=w338:dbl[])
                                n290 = Square Root(x=w338) -> (sqrt(x)=w337:dbl[])
                                n291 = Build Array (concatenate)(w337, 0.0) -> (w333:dbl[])
                                n292 = global write "G_ALL.vi" "dist lane"(w333) -> ()
                              }
                            }
                          }
                        }
                      }
                      frame #1 {
                        n293 = global read "G_ALL.vi" "x origin"() -> (w425:dbl[])
                        n294 = Empty Array?(array=w425) -> (empty?=w424:bool)
                        n295 = Or(x="lane keep", y=w424) -> (x .or. y?=w421:bool)
                        n296 = call "path steer4.vi"("lane"=w421) -> ("curve vel limit"=w422:dbl, "handle"=w420:dbl)  [unwired: 9 in]
                        n297 = global write "G_ALL.vi" "Steering"(w420) -> ()
                        n298 = global write "G_ALL.vi" "curve vel limit"(w422) -> ()
                      }
                    }
                  }
                  frame True {
                    n299 = flat-sequence {
                      tunnel: [w444] -> w429
                      tunnel: w429 -> [w472]
                      tunnel: [w472] -> w428
                      tunnel: w428 -> [w486]
                      tunnel: [w486] -> w427
                      tunnel: w427 -> [w500]
                      tunnel: [w500] -> w426
                      tunnel: w426 -> [w516]
                      frame #0 {
                        w431 = FALSE ("X Scale.Loose Fit")
                        w430 = u8 0 ("X Scale.Scale Fit")
                        n300 = call "initvar.vi"() -> ()  [unwired: 12 in]
                        n301 = property on="XY Graph" class="XYGraph (strict)"("XScale.ScaleFit"=w430, "YScale.ScaleFit"=w430, "XScale.LooseFit"=w431, "YScale.LooseFit"=w431) -> ()  [unwired: 2 in, 2 out]
                      }
                      frame #1 {
                        n302 = Bundle("Minimum"=-5.0, "Minimum"=37.3, "Minimum"=10.0, "Minimum"=1.0, "Minimum"=-20.0) -> (w436:T14)  [unwired: 1 in]
                        n303 = Bundle("Minimum"=-22.6, "Minimum"=22.6, "Minimum"=10.0, "Minimum"=1.0, "Minimum"=-20.0) -> (w443:T14)  [unwired: 1 in]
                        n304 = property on="XY Graph" class="XYGraph (strict)"("XScale.Range"=w443) -> ()  [unwired: 2 in, 2 out]
                        n305 = property on="XY Graph" class="XYGraph (strict)"("YScale.Range"=w436) -> ()  [unwired: 2 in, 2 out]
                      }
                      frame #2 {
                        n306 = global read "G_ALL.vi" "file path"() -> (w445:path)
                        n307 = Build Path(base path=w445, name or relative path="wpt") -> (appended path=w446:path)
                        n308 = call "Read From Measurement File2"("Filename"=w446, "Reset"=TRUE) -> ("error out"=w449:errorcluster, "Filename Out"=w444:path, "Signals"=w451:dynamicdata)  [unwired: 4 in, 3 out]
                        n309 = Unbundle By Name(w449) -> ("status"=w448:bool)
                        n310 = case shown="False" w448 {
                          tunnel: w451 -> [w452 _]
                          frame False {
                            n311 = call "Convert from Dynamic Data2"("Dynamic Data Type"=w452) -> ("Array"=w454:dbl[][])  [unwired: 3 in]
                            n312 = Empty Array?(array=w454) -> (empty?=w453:bool)
                            n313 = case shown="False" w453 {
                              tunnel: w454 -> [w455 _]
                              frame False {
                                n314 = global write "G_ALL.vi" "xym 1"(w455) -> ()
                                n315 = Index Array(array=w455, index (row) #1=4 ("disabled index (col)"), index (row) #2=3 ("index (col)"), index (row) #3=7 ("index (row)")) -> (element #1=w461:dbl[], element #2=w460:dbl[], element #3=w456:dbl[])  [unwired: 3 in]
                                n316 = global write "G_ALL.vi" "x origin"(w461) -> ()
                                n317 = global write "G_ALL.vi" "y origin"(w460) -> ()
                                n318 = global write "G_ALL.vi" "mission"(w456) -> ()
                              }
                              frame True {
                                w462 = dbl[] [] ("x origin")
                                n319 = global write "G_ALL.vi" "x origin"(w462) -> ()
                                n320 = global write "G_ALL.vi" "y origin"(w462) -> ()
                              }
                            }
                          }
                          frame True {
                            w463 = dbl[] [] ("x origin")
                            n321 = global write "G_ALL.vi" "x origin"(w463) -> ()
                            n322 = global write "G_ALL.vi" "y origin"(w463) -> ()
                          }
                        }
                      }
                      frame #3 {
                        n323 = global read "G_ALL.vi" "file path"() -> (w471:path)
                        n324 = Build Path(base path=w471, name or relative path="wpt") -> (appended path=w470:path)
                        n325 = call "Read From Measurement File"("Filename"=w470, "Reset"=TRUE) -> ("error out"=w467:errorcluster, "Signals"=w465:dynamicdata)  [unwired: 4 in, 4 out]
                        n326 = Unbundle By Name(w467) -> ("status"=w468:bool)
                        n327 = case shown="False" w468 {
                          tunnel: w465 -> [w474 _]
                          tunnel: [w473 _] -> w464
                          frame False {
                            n328 = call "Convert from Dynamic Data"("Dynamic Data Type"=w474) -> ("Array"=w476:dbl[][])  [unwired: 3 in]
                            n329 = Empty Array?(array=w476) -> (empty?=w475:bool)
                            n330 = case shown="False" w475 {
                              tunnel: w476 -> [w477 _]
                              tunnel: [w477 _] -> w473
                              frame False {
                              }
                              frame True {
                              }
                            }
                          }
                          frame True {
                          }
                        }
                        n331 = global write "G_ALL.vi" "xym 2"(w464) -> ()
                      }
                      frame #4 {
                        n332 = global read "G_ALL.vi" "file path"() -> (w479:path)
                        n333 = Build Path(base path=w479, name or relative path="wpt") -> (appended path=w480:path)
                        n334 = call "Read From Measurement File3"("Filename"=w480, "Reset"=TRUE) -> ("error out"=w483:errorcluster, "Signals"=w485:dynamicdata)  [unwired: 4 in, 4 out]
                        n335 = Unbundle By Name(w483) -> ("status"=w482:bool)
                        n336 = case shown="False" w482 {
                          tunnel: w485 -> [w488 _]
                          tunnel: [w487 _] -> w478
                          frame False {
                            n337 = call "Convert from Dynamic Data3"("Dynamic Data Type"=w488) -> ("Array"=w490:dbl[][])  [unwired: 3 in]
                            n338 = Empty Array?(array=w490) -> (empty?=w489:bool)
                            n339 = case shown="False" w489 {
                              tunnel: w490 -> [w491 _]
                              tunnel: [w491 _] -> w487
                              frame False {
                              }
                              frame True {
                              }
                            }
                          }
                          frame True {
                          }
                        }
                        n340 = global write "G_ALL.vi" "xym 3"(w478) -> ()
                      }
                      frame #5 {
                        n341 = global read "G_ALL.vi" "file path"() -> (w499:path)
                        n342 = Build Path(base path=w499, name or relative path="wpt") -> (appended path=w498:path)
                        n343 = call "Read From Measurement File4"("Filename"=w498, "Reset"=TRUE) -> ("error out"=w495:errorcluster, "Signals"=w493:dynamicdata)  [unwired: 4 in, 4 out]
                        n344 = Unbundle By Name(w495) -> ("status"=w496:bool)
                        n345 = case shown="False" w496 {
                          tunnel: w493 -> [w502 _]
                          tunnel: [w501 _] -> w492
                          frame False {
                            n346 = call "Convert from Dynamic Data4"("Dynamic Data Type"=w502) -> ("Array"=w504:dbl[][])  [unwired: 3 in]
                            n347 = Empty Array?(array=w504) -> (empty?=w503:bool)
                            n348 = case shown="False" w503 {
                              tunnel: w504 -> [w505 _]
                              tunnel: [w505 _] -> w501
                              frame False {
                              }
                              frame True {
                              }
                            }
                          }
                          frame True {
                          }
                        }
                        n349 = global write "G_ALL.vi" "xym 4"(w492) -> ()
                      }
                      frame #6 {
                        n350 = Strip Path(path=w516) -> (name=w512:string)  [unwired: 1 out]
                        n351 = local write "Load Path"(FALSE ("Load WPT")) -> ()
                        n352 = local write "reset path"(TRUE ("reset path")) -> ()
                        n353 = Match Pattern(string=w512, regular expression="_") -> (after substring=w514:string)  [unwired: 1 in, 3 out]
                        n354 = Match Pattern(string=w514, regular expression=".lvm") -> (before substring=w511:string)  [unwired: 1 in, 3 out]
                        n355 = Scan From String(input string=w511, default 1=T13."KAIST" ("map name")) -> (error out=w510:errorcluster, output 1=w508:T13)  [unwired: 3 in, 2 out]
                        n356 = case shown="Error" w510 {
                          tunnel: [w521 w522] -> w509
                          tunnel: w508 -> [w521 _]
                          frame No Error {
                          }
                          frame Error {
                            n357 = global read "G_ALL.vi" "GPSDATA"() -> (w523:T15)
                            n358 = Unbundle By Name(w523) -> ("map_idx"=w522:i32)
                          }
                        }
                        n359 = call "mapconf.vi"("map name"=w509) -> ("y"=w518:cluster{dbl, dbl, "y":dbl, "y":dbl, dbl}, "x"=w519:cluster{dbl, dbl, "y":dbl, "y":dbl, dbl}, "new picture"=w520:picture)  [unwired: 8 in]
                        n360 = property on="XY Graph 2" class="XYGraph (strict)"("PlotImages.Back"=w520) -> ()  [unwired: 2 in, 2 out]
                        n361 = property on="XY Graph 2" class="XYGraph (strict)"("XScale.Range"=w519, "YScale.Range"=w518) -> ()  [unwired: 2 in, 2 out]
                      }
                    }
                  }
                }
              }
              frame True {
                n362 = flat-sequence {
                  tunnel: [w527] -> w524
                  tunnel: w524 -> [w595]
                  frame #0 {
                    w525 = 0.0
                    n363 = global write "G_ALL.vi" "VS_des"(w525) -> ()
                    n364 = global write "G_ALL.vi" "Steering"(w525) -> ()
                  }
                  frame #1 {
                    n365 = local read "Make WPT"() -> (w526:bool)
                    n366 = Initialize Array(0.0 ("element"), 7 ("dimension size"), 1 ("dimension size")) -> (w528:dbl[][])
                    n367 = while {
                      shift-right: [w532] -> w527
                      shift-left: w528 -> [w534]
                      shift-right: [FALSE] -> _
                      shift-left: w526 -> [w535]
                      stop <- w537 stop-if-true
                      n368 = flat-sequence {
                        tunnel: [w549] -> w533
                        frame #0 {
                          n369 = global read "G_ALL.vi" "GPSDATA"() -> (w544:T15)
                          n370 = global read "G_ALL.vi" "CARDATA"() -> (w543:T7)
                          n371 = Unbundle By Name(w544) -> ("lat"=w548:dbl, "lon"=w547:dbl, "hgt"=w546:dbl, "map_idx"=w542:i32)
                          n372 = Unbundle By Name(w543) -> ("y"=w540:dbl, "x"=w539:dbl, "VS_can"=w541:dbl)
                          n373 = To Double Precision Float(number=w542) -> (double precision float=w545:dbl)
                          n374 = Build Array(w548, w547, w546, w540, w539, w546, w541, w545) -> (w549:dbl[])
                        }
                      }
                      n375 = local read "Make WPT"() -> (w538:bool)
                      n376 = Not(x=w538) -> (.not. x?=w537:bool)
                      n377 = case shown="False" w535 {
                        tunnel: w534 -> [w564 w581]
                        tunnel: w533 -> [w563 w579]
                        tunnel: [w562 w578] -> w532
                        frame False {
                          n378 = Array Size(array=w564) -> (size(s)=w572:i32[])
                          n379 = Index Array(array=w563, index #1=3 ("index"), index #2=4 ("index")) -> (element #1=w558:dbl, element #2=w556:dbl)
                          n380 = Index Array(array=w572, index=1) -> (element=w561:i32)
                          n381 = Decrement(x=w561) -> (x-1=w560:i32)
                          n382 = Index Array(array=w564, index (col)=w560) -> (element=w568:dbl[])  [unwired: 1 in]
                          n383 = Index Array(array=w568, index #1=3 ("index"), index #2=4 ("index")) -> (element #1=w559:dbl, element #2=w557:dbl)
                          n384 = Subtract(x=w559, y=w558) -> (x-y=w555:dbl)
                          n385 = Subtract(x=w557, y=w556) -> (x-y=w554:dbl)
                          n386 = Square(x=w555) -> (x^2=w553:dbl)
                          n387 = Square(x=w554) -> (x^2=w552:dbl)
                          n388 = Add(x=w553, y=w552) -> (x+y=w551:dbl)
                          n389 = Greater Or Equal?(x=w551, y=0.25) -> (x >= y?=w565:bool)
                          n390 = case shown="True" w565 {
                            tunnel: w564 -> [w573 w577]
                            tunnel: w561 -> [_ w574]
                            tunnel: w563 -> [_ w576]
                            tunnel: [w573 w575] -> w562
                            frame False {
                            }
                            frame True {
                              n391 = Insert Into Array(array=w577, index (col)=w574, new element=w576) -> (w575:dbl[][])  [unwired: 1 in]
                            }
                          }
                        }
                        frame True {
                          n392 = Replace Array Subset(array=w581, new element=w579, index (col)=0 ("disabled index (col)")) -> (w578:dbl[][])  [unwired: 1 in]
                        }
                      }
                    }
                  }
                  frame #2 {
                    n393 = call "Convert to Dynamic Data"("2D Array"=w595) -> ("Dynamic Data Type"=w596:dynamicdata)  [unwired: 3 in]
                    n394 = global read "G_ALL.vi" "GPSDATA"() -> (w585:T15)
                    n395 = Unbundle By Name(w585) -> ("map_idx"=w583:i32)
                    n396 = Get Date/Time In Seconds() -> (seconds since 1Jan1904=w593:timestamp)
                    n397 = Format Date/Time String(time format string (%c)="%2y%2m%2d%2H%2M", seconds (now)=w593) -> (date/time string=w591:string)  [unwired: 1 in]
                    n398 = Format Into String(w583) -> (resulting string=w582:string)  [unwired: 3 in, 1 out]
                    n399 = global read "G_ALL.vi" "file path"() -> (w584:path)
                    n400 = Build Path(base path=w584, name or relative path="wpt") -> (appended path=w588:path)
                    n401 = Concatenate Strings(w591, "_" ("string"), w582, ".lvm" ("string")) -> (w587:string)
                    n402 = Build Path(base path=w588, name or relative path=w587) -> (appended path=w586:path)
                    n403 = call "save wpt"("Signals"=w596, "Reset"=TRUE, "Filename"=w586) -> ()  [unwired: 14 in, 3 out]
                  }
                }
              }
            }
          }
        }
      }
    }
  }
  n404 = flat-sequence {
    frame #0 {
      # "Sensor paser"
    }
    frame #1 {
      w598 = dbl[][] [] ("M_lane_left")
      w599 = dbl[] [] ("M_lane_left")
      n405 = local write "Log"(FALSE ("obs")) -> ()
      n406 = global write "G_SEN.vi" "sensor_obs"(w598) -> ()
      n407 = global write "G_SEN.vi" "sensor_lane"(w598) -> ()
      n408 = global write "G_SEN.vi" "M_lane_left"(w599) -> ()
      n409 = global write "G_SEN.vi" "M_lane_right"(w599) -> ()
      n410 = global write "G_SEN.vi" "M_lane_center"(w599) -> ()
    }
    frame #2 {
      n411 = while {
        stop <- FALSE ("Loop 4") stop-if-true
        n412 = flat-sequence {
          frame #0 {
            n413 = disable-structure shown="Enabled" {
              disable-tunnel: [w605 w607] -> w602
              frame Disabled {
                n414 = Wait Until Next ms Multiple(millisecond multiple=u32 10 ("milliseconds to wait")) -> (millisecond timer value=w605:u32)
              }
              frame Enabled {
                n415 = Tick Count (ms)() -> (millisecond timer value=w607:u32)
              }
            }
            n416 = feedback #5() -> (w604:u32)  [unwired: 1 in]
            n417 = feedback-in #5(w602) -> ()
            n418 = Subtract(x=w602, y=w604) -> (x-y=→"sensor":u32)
          }
          frame #1 {
            n419 = disable-structure shown="Enabled" {
              frame Enabled {
                w609 = 0.0 ("roll")
                n420 = local read "Velodyne"() -> (w610:T1)
                n421 = call "velosterpaser384.vi"("roll"=w609, "pitch"=w609, "heading"=w609, "dX"=w609, "dY"=w609, "dZ"=w609, "Velodyne"=w610) -> ()  [unwired: 12 in, 1 out]
              }
              frame Disabled {
                n422 = call "velosterpaserraw.vi"() -> ()  [unwired: 20 in]
              }
            }
            n423 = global read "G_LCM.vi" "Mobileye name"() -> (w608:string)
            n424 = case shown="\"vision_lane_pt\"" w608 {
              frame Default {
                n425 = call "mobileyelanepaser4.vi"("count hold"=u64 15, "thresh  c"=0.5, "thresh  b"=0.06 ("thresh 2"), "thresh r"=0.009 ("y")) -> ()  [unwired: 4 in, 4 out]
                n426 = call "mobileyepaser.vi"() -> ()  [unwired: 11 in, 1 out]
              }
              frame "vision_lane_pt" {
                n427 = flat-sequence {
                  frame #0 {
                    n428 = disable-structure shown="Disabled" {
                      frame Disabled {
                        n429 = call "laneleftright.vi"() -> ()  [unwired: 10 in, 2 out]
                      }
                      frame Enabled {
                      }
                    }
                  }
                  frame #1 {
                    n430 = call "laneleftright2.vi"() -> ()  [unwired: 10 in, 2 out]
                  }
                }
              }
              frame "Mobileye560_temp" {
                n431 = global read "G_LCM.vi" "Mobileye_RAW_SNAP"() -> (w619:T17)
                n432 = Unbundle By Name(w619) -> ("sys time"=w617:i64, "size"=w620:i32, "data"=w621:u8[])
                n433 = feedback-in #6(w617) -> ()
                n434 = feedback #6(i64 -1 ("sys time")) -> (w616:i64)
                n435 = case shown="False" TRUE {
                  selector: TRUE -> [w622 _]
                  tunnel: w621 -> [_ w626]
                  tunnel: w620 -> [_ w623]
                  frame False {
                    n436 = global write "G_SEN.vi" "M_lane_update"(w622) -> ()
                  }
                  frame True {
                    n437 = Divide(x=w623, y=16) -> (x/y=w625:dbl)
                    n438 = for {
                      N: w625 -> [_]
                      tunnel: w626 -> [w647]
                      i -> [w646]
                      w639 = 4 ("length")
                      w637 = 8 ("index")
                      w645 = 16 ("y")
                      n439 = Multiply(x=w646, y=w645) -> (x*y=w644:i32)
                      n440 = Array Subset(array=w647, index=w644, length=w645) -> (w629:u8[])
                      n441 = Delete From Array(array=w629, length=w637, index=w637) -> (deleted portion=w630:u8[], array with subset deleted=w638:u8[])
                      n442 = Delete From Array(array=w638, length=w639, index=w639) -> (deleted portion=w643:u8[], array with subset deleted=w640:u8[])
                      n443 = Type Cast(type=u32 0, x=w640) -> (*(type *) &x=w631:u32)
                      n444 = Type Cast(type=u32 0, x=w643) -> (*(type *) &x=w632:u32)
                      n445 = Multiply(x=w632, y=1e-07) -> (x*y=w635:dbl)
                      n446 = To Time Stamp(1:w635) -> (0:w634:timestamp)
                      n447 = Bundle By Name(cluster=T16 {"identifier"=0, "timestamp"=timestamp(0 s since 1904-01-01), "payload"=[]} ("can cluster"), "identifier"=w631, "payload"=w630, "timestamp"=w634) -> (w628:T16)
                      n448 = call "mobileye_decoder_PC.vi"("can cluster"=w628, "name"="Mobileye560") -> ()  [unwired: 10 in]
                    }
                  }
                }
                n449 = Not Equal?(x=w617, y=w616) -> ()  [unwired: 1 out]
              }
              frame "Mobileye560S" {
                n450 = global read "G_LCM.vi" "Mobileye_RAW_SNAP"() -> (w650:T17)
                n451 = Unbundle By Name(w650) -> ("data"=w649:u8[])
                n452 = Byte Array To String(unsigned byte array=w649) -> (string=w648:string)
                n453 = while {
                  shift-right: [w653] -> _
                  shift-left: w648 -> [w655]
                  stop <- w654 stop-if-true
                  w659 = "S" ("regular expression")
                  n454 = Match Pattern(string=w655, regular expression="S") -> (after substring=w668:string)  [unwired: 1 in, 3 out]
                  n455 = Match Pattern(string=w668, regular expression=" ") -> (before substring=w666:string, after substring=w664:string)  [unwired: 1 in, 2 out]
                  n456 = Hexadecimal String To Number(string=w666) -> (number=w657:u32)  [unwired: 2 in, 1 out]
                  n457 = Match Pattern(string=w664, regular expression=w659) -> (before substring=w663:string, match substring=w660:string, after substring=w661:string)  [unwired: 1 in, 1 out]
                  n458 = Not Equal?(x=w660, y=w659) -> (x != y?=w654:bool)
                  n459 = Concatenate Strings(w660, w661) -> (w653:string)
                  n460 = for {
                    N: 8 -> [_]
                    tunnel: w663 -> [w677]
                    tunnel: [w673] -> w656 mode=indexing
                    i -> [w672]
                    n461 = Multiply(x=2, y=w672) -> (x*y=w675:i32)
                    n462 = String Subset(string=w677, offset (0)=w675, length (rest)=2 ("length (rest)")) -> (substring=w670:string)
                    n463 = Hexadecimal String To Number(string=w670, default (0uL)=u8 0) -> (number=w673:u8)  [unwired: 1 in, 1 out]
                  }
                  n464 = Get Date/Time In Seconds() -> (seconds since 1Jan1904=w662:timestamp)
                  n465 = Bundle By Name(cluster=T16 {"identifier"=0, "timestamp"=timestamp(0 s since 1904-01-01), "payload"=[]} ("can cluster"), "identifier"=w657, "payload"=w656, "timestamp"=w662) -> (w651:T16)
                  n466 = call "mobileye_decoder_PC.vi"("can cluster"=w651, "name"="Mobileye560") -> ()  [unwired: 10 in]
                }
              }
            }
          }
          frame #2 {
            w680 = TRUE ("Sensor [F12]")
            n467 = global read "G_LCM.vi" "Mobileye name"() -> (w678:string)
            n468 = call "Ibeopaser.vi"("theta"=-2.5, "Hide Transparent"=w680, "Sensor [F12]"=w680) -> ("x_sensor"=w684:cluster{"idx":i32, "x":dbl, "y":dbl, "h":dbl}, "etc"=w682:dbl[][], "lane"=w683:dbl[][], "obs"=w685:dbl[][], "update"=w681:bool)  [unwired: 4 in]
            n469 = case shown="True" w681 {
              tunnel: w685 -> [_ w693]
              tunnel: w684 -> [_ w688]
              tunnel: w683 -> [_ w690]
              tunnel: w682 -> [_ w691]
              frame False {
              }
              frame True {
                n470 = disable-structure shown="Enabled" {
                  disable-tunnel: w693 -> [w698 w700]
                  disable-tunnel: [w697 w700] -> w692
                  disable-tunnel: w691 -> [w696 _]
                  disable-tunnel: w690 -> [w695 w699]
                  disable-tunnel: [w694 w699] -> w689
                  frame Disabled {
                    n471 = call "test3.vi"("sensor_all"=w696, "sensor_lane"=w695, "sensor_obs"=w698) -> ("lane"=w694:dbl[][], "obs"=w697:dbl[][])  [unwired: 6 in, 1 out]
                  }
                  frame Enabled {
                  }
                }
                n472 = global write "G_ALL.vi" "x_ibeo"(w688) -> ()
                n473 = global write "G_SEN.vi" "sensor_obs"(w692) -> ()
                n474 = global write "G_SEN.vi" "sensor_lane"(w689) -> ()
              }
            }
            n475 = case shown="Default" w678 {
              frame Default {
                n476 = global read "G_SEN.vi" "M_lane_update"() -> (w686:bool)
                n477 = local write "lane update"(w686) -> ()
              }
              frame "vision_lane_pt" {
                n478 = global write "G_SEN.vi" "M_lane_update"("lane update") -> ()
              }
            }
          }
          frame #3 {
            n479 = disable-structure shown="Enabled" {
              frame Disabled {
                n480 = global read "G_ALL.vi" "x_ibeo"() -> (w702:cluster{"idx":i32, "x":dbl, "y":dbl, "h":dbl})
                n481 = disable-structure shown="Disabled" {
                  disable-tunnel: [w729 w763] -> w703
                  disable-tunnel: w702 -> [w715 w762]
                  disable-tunnel: [w714 w762] -> w701
                  frame Disabled {
                    n482 = global read "G_ALL.vi" "CARDATA"() -> (w716:T7)
                    n483 = global read "G_SEN.vi" "Lane_R_M"() -> (w738:dbl[])
                    n484 = global read "G_SEN.vi" "Lane_L_M"() -> (w735:dbl[])
                    n485 = Unbundle By Name(w716) -> ("x"=w713:dbl, "y"=w712:dbl, "heading"=w711:dbl)
                    n486 = Index Array(array=w738, index=0) -> (element=w740:dbl)
                    n487 = Index Array(array=w735, index=0) -> (element=w733:dbl)
                    n488 = Bundle By Name(cluster=w715, "x"=w713, "y"=w712, "h"=w711) -> (w714:cluster{"idx":i32, "x":dbl, "y":dbl, "h":dbl})
                    n489 = Greater?(x=w740, y=0.65) -> (0:w739:bool)
                    n490 = Greater?(x=w733, y=0.65) -> (0:w734:bool)
                    n491 = case shown="True" w739 {
                      tunnel: w738 -> [_ w753]
                      tunnel: [_ w754] -> w724
                      tunnel: [_ w752] -> w723
                      frame False {
                      }
                      frame True {
                        n492 = global read "G_SEN.vi" "y_mobileye"() -> (w752:dbl[])
                        n493 = Index Array(array=w753, index #1=1 ("index")) -> (element #1=w759:dbl, element #2=w758:dbl, element #3=w755:dbl)  [unwired: 2 in]
                        n494 = Square(x=w752) -> (x^2=w760:dbl[])
                        n495 = Multiply(x=w758, y=w752) -> (x*y=w756:dbl[])
                        n496 = Multiply(x=w759, y=w760) -> (x*y=w757:dbl[])
                        n497 = Compound Arithmetic op=ADD(w757, w756, w755) -> (w754:dbl[])
                      }
                    }
                    n498 = case shown="True" w734 {
                      tunnel: w735 -> [_ w743]
                      tunnel: [_ w744] -> w722
                      tunnel: [_ w742] -> w721
                      frame False {
                      }
                      frame True {
                        n499 = global read "G_SEN.vi" "y_mobileye"() -> (w742:dbl[])
                        n500 = Index Array(array=w743, index #1=1 ("index")) -> (element #1=w749:dbl, element #2=w748:dbl, element #3=w745:dbl)  [unwired: 2 in]
                        n501 = Square(x=w742) -> (x^2=w750:dbl[])
                        n502 = Multiply(x=w748, y=w742) -> (x*y=w746:dbl[])
                        n503 = Multiply(x=w749, y=w750) -> (x*y=w747:dbl[])
                        n504 = Compound Arithmetic op=ADD(w747, w746, w745) -> (w744:dbl[])
                      }
                    }
                    n505 = Build Array(w724, w723) -> (w728:dbl[][])
                    n506 = Build Array(w722, w721) -> (w726:dbl[][])
                    n507 = Array Subset(array=w728, index (col)=0 ("index"), length (col)=5 ("length")) -> (w727:dbl[][])  [unwired: 2 in]
                    n508 = Array Subset(array=w726, index (col)=0 ("index"), length (col)=5 ("length")) -> (w725:dbl[][])  [unwired: 2 in]
                    n509 = Transpose 2D Array(2D array=w727) -> (transposed array=w731:dbl[][])
                    n510 = Transpose 2D Array(2D array=w725) -> (transposed array=w730:dbl[][])
                    n511 = Build Array (concatenate)(w731, w730) -> (w729:dbl[][])
                  }
                  frame Enabled {
                    n512 = global read "G_SEN.vi" "sensor_obs"() -> (w763:dbl[][])
                  }
                }
                n513 = global read "G_SEN.vi" "sensor_obs_log"() -> (w707:dbl[][])
                n514 = call "sensor_log2.vi"("xmax"=999999999.0, "FF"=1.0 ("t"), "xmin"=-99999999.0, "x_sensor"=w701, "ymin"=-99999999.0, "ymax"=99999999.0, "sensor_log in"=w707, "sensor_obs"=w703) -> ("sensor_log out"=w706:dbl[][])  [unwired: 3 in]
                n515 = global write "G_SEN.vi" "sensor_obs_log"(w706) -> ()
              }
              frame Enabled {
                n516 = case shown="True" "Log" {
                  frame False {
                    n517 = disable-structure shown="Enabled" {
                      frame Enabled {
                        n518 = global write "G_SEN.vi" "sensor_obs_log"(dbl[][] [] ("sensor_obs_log")) -> ()
                      }
                      frame Disabled {
                      }
                    }
                  }
                  frame True {
                    n519 = global read "G_ALL.vi" "CARDATA"() -> (w766:T7)
                    n520 = Unbundle By Name(w766) -> ("VS_can"=w768:dbl)
                    n521 = Not Equal To 0?(x=w768) -> (x != 0?=w767:bool)
                    n522 = case shown="True" w767 {
                      frame False {
                      }
                      frame True {
                        n523 = global read "G_SEN.vi" "sensor_obs_log"() -> (w772:dbl[][])
                        n524 = global read "G_SEN.vi" "sensor_obs"() -> (w773:dbl[][])
                        n525 = global read "G_ALL.vi" "x_ibeo"() -> (w769:cluster{"idx":i32, "x":dbl, "y":dbl, "h":dbl})
                        n526 = call "sensor_log2.vi"("xmax"=5.0, "FF"=0.99 ("t"), "xmin"=-5.0, "x_sensor"=w769, "ymin"=0.0, "ymax"=15.0, "sensor_log in"=w772, "sensor_obs"=w773) -> ("sensor_log out"=w771:dbl[][])  [unwired: 3 in]
                        n527 = global write "G_SEN.vi" "sensor_obs_log"(w771) -> ()
                      }
                    }
                  }
                }
              }
            }
          }
        }
      }
    }
  }
